vi "Process.vi"(8 "error in":errorcluster, 11 "Control Experiment":refnum<class "SMO.Control Experiment.lvclass">) -> (0 "error out":errorcluster, 3 "Control Experiment out":refnum<class "SMO.Control Experiment.lvclass">)   [LabVIEW 2019, in "SMO.Control Experiment.lvclass"]
doc: "---------------------------------------------------------------\nJKI State Machine Objects™\nhttp://jki.net/state-machine-objects/\nCopyright (C) 2005-2015, JKI <info@jki.net>\nALL RIGHTS RESERVED"
uses:
  SMO.Control Experiment.lvclass
  C:/Program Files (x86)/National Instruments/LabVIEW 2019/vi.lib/JKI/JKI SMO/SMO/SMO.lvclass
  C:/Program Files (x86)/National Instruments/LabVIEW 2019/user.lib/LevyLab/Instrument Framework/SMOs/Instrument/Instrument.lvclass
  <userlib>/LevyLab/Instrument Framework/SMOs/Configuration/Configuration.lvclass
  SMO.Control Experiment UI/Typedefs/UI Config--Cluster.ctl
  SMO.Control Experiment UI/Typedefs/UI Channels--Cluster.ctl
  SMO.Control Experiment UI/Typedefs/UI Channels.AI--Cluster.ctl
  SMO.Control Experiment UI/Typedefs/UI Channels.Device--Cluster.ctl
  Control Experiment/Typedefs/KH Mode-enum.ctl
  SMO.Control Experiment UI/Typedefs/UI Channels.KH--Cluster.ctl
  <userlib>/LevyLab/Krohn Hite 7008/typedefs/Input Configuration-Enum.ctl
  <userlib>/LevyLab/Krohn Hite 7008/typedefs/Gain-Enum.ctl
  <userlib>/LevyLab/Krohn Hite 7008/typedefs/Shunt-Enum.ctl
  SMO.Control Experiment UI/Typedefs/UI Channels.AO--Cluster.ctl
  Control Experiment/Typedefs/Instrument--enum.ctl
  <userlib>/LevyLab/Krohn Hite 7008/typedefs/Coupling-Enum.ctl
  <userlib>/LevyLab/Krohn Hite 7008/typedefs/Filter-Enum.ctl
  SMO.Control Experiment UI/Typedefs/KH Cluster--Cluster.ctl
  <userlib>/LevyLab/Krohn Hite 7008/typedefs/SetAll-Cluster.ctl
  <userlib>/LevyLab/Krohn Hite 7008/typedefs/Channel-Enum.ctl
  SMO.Control Experiment.lvclass/SMO.Control Experiment.ctl
  <vilib>/JKI/JKI SMO/SMO/SMO.lvclass/SMO.ctl
  <vilib>/Utility/sysdir.llb/System Directory Type.ctl
  Control Experiment/Typedefs/Experiment Description--cluster.ctl
  Control Experiment/Typedefs/Instrument Types--combo.ctl
  Control Experiment/Control Experiment.lvclass/Control Experiment.ctl
  Control Experiment/Typedefs/Wiring Description--v2--cluster.ctl
  Control Experiment/Typedefs/Control Experiment JSON--cluster.ctl
  <userlib>/LevyLab/Krohn Hite 7008/Instrument.KH7008.lvclass/Instrument.KH7008.ctl
  c232f248-acab-4811-9a90-d7a35ba50f8f.vi
  <vilib>/JKI/JKI SMO/SMO/Private/ReftoDVR--SMO.vi
  <vilib>/JDP Science/JSONtext/Variant to JSON Text.vi
  <vilib>/JDP Science/JSONtext/LVClass Serializer/JSONtext LVClass Serializer.lvclass
  <userlib>/LevyLab/Instrument Framework/SMOs/Instrument/Instrument.lvclass
  <userlib>/LevyLab/Krohn Hite 7008/Instrument.KH7008.lvclass
  <userlib>/LevyLab/Lockin-Multichannel/Instrument.Lockin/Instrument.Lockin.lvclass
  <userlib>/LevyLab/Instrument Framework/Instrument Types/Strain/Instrument.Strain.lvclass
  <userlib>/LevyLab/Instrument Framework/Instrument Types/CBridge/Instrument.CBridge.lvclass
  <vilib>/JKI/JKI SMO/SMO/SMO.lvclass
  Control Experiment/Control Experiment.lvclass
  SMO.Control Experiment UI/SMO.Control Experiment UI.lvclass
panel:
  # "Instrument.\nControl Experiment\nBackend"
  # "For instructions on how to use the JKI State Machine Objects, examples and video tutorials, visit:\nhttp://jki.net/state-machine-objects/\n\nJKI State Machine Objects™\nhttp://jki.net/state-machine-objects/\nCopyright (C) 2005-2015, JKI <info@jki.net>\nALL RIGHTS RESERVED"
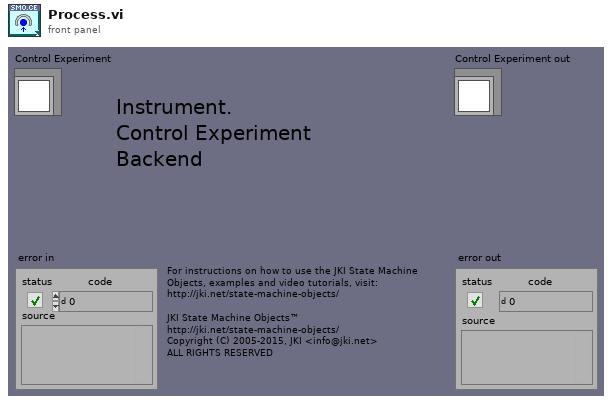
[diagram p1: front panel]
types:
  T1 = enum32{"invalid app kind", "Development System", "Run Time System", "Student Edition", "Embedded LabVIEW", "Evaluation", "Custom"}
  T2 = enum32{"Invalid", "Standard", "Closed", "Hidden", "Minimized", "Maximized"}
  T3 = enum32{"Bad", "Idle", "Run top level", "Running"}
  T4 = typedef "Control Experiment.lvclass/Experiment Description--cluster.ctl" = cluster{"User":string, "Device":string, "Device Path":path, "Device Description":string, "Experiment Path":path, "Experiment Description":string, "Instrument":T5, "Instruments":cluster{"class path":path, "Address":string, "Type":T6}[], "Sweep":cluster{"key":string, "value":variant}[]}
  T5 = typedef "Control Experiment.lvclass/Instrument--enum.ctl" = enum16{"----- AFM/EBL -----", "AGILENT", "CYPHER", "Gemini2", "JEOL", "MFP3D", "----- Cryostat -----", "CF900", "DR200", "MNK", "PPMS (simulated)", "PPMS 1", "PPMS 2", "PPMS 3", "----- Optics -----", "THz 1 (Element 2/Montana)", "THz 2 (Tsunami/Janis)"}
  T6 = typedef "Control Experiment.lvclass/Instrument Types--combo.ctl" = string
  T7 = typedef "Control Experiment.lvclass/Wiring Description--v2--cluster.ctl" = cluster{"AI":cluster{"Channel":u32, "Gain":dbl}, "Device":cluster{"Electrode":string, "Label":string, "Type":string}, "KH":cluster{"Channel":string, "Configuration":string, "Gain":u32, "Shunt Resistor":u32}, "AO":cluster{"Channel":u32, "Gain":dbl}}
  T8 = typedef "SMO.Control Experiment.lvclass/PrivateEvents--Control Experiment.saveKHpreset.ctl" = string
  T9 = typedef "SMO.Control Experiment.lvclass/PrivateEvents--Control Experiment.loadKHpreset.ctl" = string
  T10 = typedef "SMO.Control Experiment.lvclass/UI Config--Cluster.ctl" = cluster{"Metadata":cluster{"Sample (SAXXXX)":string, "Device (YYYYMMDD)":string, "Description":string, "Username":string, "Default Path":path}, "Number of AI":i32, "UI Channels []":T11[], "Instruments":cluster{"Lockin Address":string, "Krohn Hite?":bool, "KH Addresses":refnum<visa-resource-name>[], "Strain Cell?":bool, "Strain Cell Address":refnum<visa-resource-name>, "C Bridge?":bool, "Capacitance Bridge Address":refnum<visa-resource-name>, "Instrument":T5}, "Krohn Hite":cluster{"Defualt Shunt Resistor":T18, "Default Gain":T17, "Coupling":T20, "Bandwidth Filter":T21}}
  T11 = typedef "SMO.Control Experiment UI.lvclass/UI Channels--Cluster.ctl" = cluster{"AI":T12, "Device":T13, "KH":T15, "AO":T19}
  T12 = typedef "SMO.Control Experiment UI.lvclass/UI Channels.AI--Cluster.ctl" = cluster{"Channel":u32, "Gain":dbl}
  T13 = typedef "SMO.Control Experiment UI.lvclass/UI Channels.Device--Cluster.ctl" = cluster{"Electrode":string, "Configuration":T14, "Label":u16}
  T14 = typedef "Control Experiment.lvclass/KH Mode-enum.ctl" = enum16{"Ground", "Current", "Voltage (SE)", "Voltage (Diff)", "Gate"}
  T15 = typedef "SMO.Control Experiment UI.lvclass/UI Channels.KH--Cluster.ctl" = cluster{"Channel":u16, "Configuration":T16, "Gain":T17, "Shunt Resistor":T18}
  T16 = typedef "Instrument.KH7008.lvclass/Input Configuration-Enum.ctl" = enum16{"Ground", "SE+ (-gnd)", "SE- (+gnd)", "Differential"}
  T17 = typedef "Instrument.KH7008.lvclass/Gain-Enum.ctl" = enum16{"1x", "10x", "100x", "1000x"}
  T18 = typedef "Instrument.KH7008.lvclass/Shunt-Enum.ctl" = enum16{"Open", "50 Ohms", "500 Ohms", "5k Ohms", "50k Ohms", "10M Ohm"}
  T19 = typedef "SMO.Control Experiment UI.lvclass/UI Channels.AO--Cluster.ctl" = cluster{"Channel":u32, "Gain":dbl}
  T20 = typedef "Instrument.KH7008.lvclass/Coupling-Enum.ctl" = enum16{"AC", "DC"}
  T21 = typedef "Instrument.KH7008.lvclass/Filter-Enum.ctl" = enum16{"OFF", "ON"}
  T22 = typedef "SMO.Control Experiment UI.lvclass/KH Cluster--Cluster.ctl" = cluster{"VISA Resource Name":refnum<visa-resource-name>, "KH Ch Array":T23[]}[]
  T23 = typedef "Instrument.KH7008.lvclass/SetAll-Cluster.ctl" = cluster{"Channel":T24, "Gain":T17, "Bandwidth Filter":T21, "Shunt Resistor":T18, "Coupling":T20, "Input Config":T16}
  T24 = typedef "Instrument.KH7008.lvclass/Channel-Enum.ctl" = enum16{"Channel 1", "Channel 2", "Channel 3", "Channel 4", "Channel 5", "Channel 6", "Channel 7", "Channel 8"}
  T25 = cluster{"Core":cluster{"Current VI Reference":refnum<vi>, "Close Panel on Exit?":bool, "error":errorcluster}, "Self Reference":refnum<class "SMO.Control Experiment.lvclass">, "C.E.":refnum<class "Control Experiment.lvclass">, "Config":refnum<class "Configuration.lvclass">, "UI Config":T10, "KH Cluster":T22}
  T26 = cluster{"Current VI Reference":refnum<vi>, "Close Panel on Exit?":bool, "error":errorcluster}
  T27 = typedef "SMO.lvclass/Protected Events.ctl" = cluster{"StopProcesses":refnum<user-event>, "AbortProcesses":refnum<user-event>, "Config Changed":refnum<user-event>, "Dependency":refnum<user-event>}
  T28 = typedef "SMO.Control Experiment.lvclass/PrivateEvents--Cluster.ctl" = cluster{"saveKHpreset":refnum<user-event>, "setUIconfig":refnum<user-event>, "loadKHpreset":refnum<user-event>}
  T29 = typedef "System Directory Type.ctl" = i32
  T30 = typedef "Control Experiment.lvclass/Control Experiment JSON--cluster.ctl" = cluster{"Device":cluster{"Device":string, "User":string, "Time":string, "Computer Name":string}, "Wiring":cluster{"Lockin Ch":u32[], "KH Electrodes":string[], "KH Labels":string[], "Other Electrodes":string[], "Other Labels":string[]}}
  T31 = typedef "Control Experiment.lvclass/Instruments--cluster.ctl" = cluster{"KH7008":refnum<class "Instrument.KH7008.lvclass">[], "Lockin":refnum<class "Instrument.Lockin.lvclass">, "Temperature":refnum<class "Instrument.Cryostat.lvclass">, "Magnet":refnum<class "Instrument.Cryostat.lvclass">, "Rotator":refnum<class "Instrument.Cryostat.lvclass">, "Level":refnum<class "Instrument.Cryostat.lvclass">, "Capacitance Bridge":refnum<class "Instrument.CBridge.lvclass">, "Delay Line":refnum<class "Instrument.DelayLine.lvclass">, "Strain Cell":refnum<class "Instrument.Strain.lvclass">, "VNA":refnum<class "Instrument.VNA.lvclass">, "Voltage Source":refnum<class "Instrument.VSource.lvclass">}
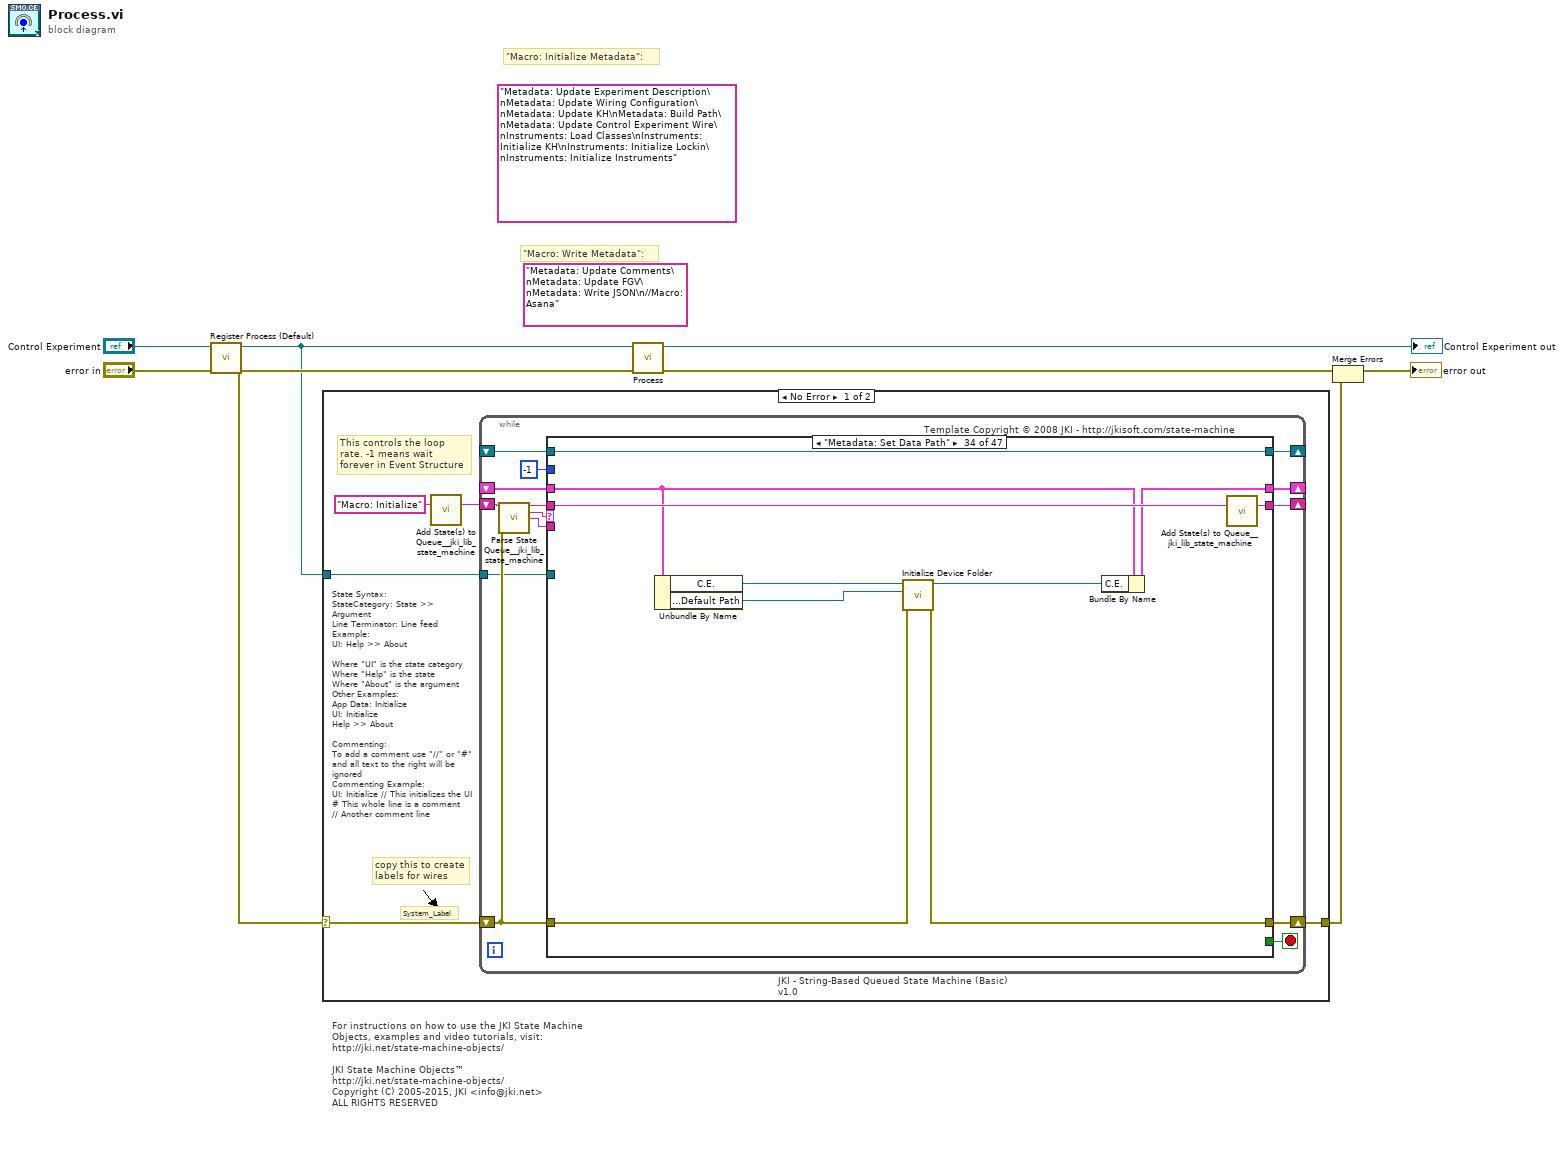
[diagram p0: block diagram]
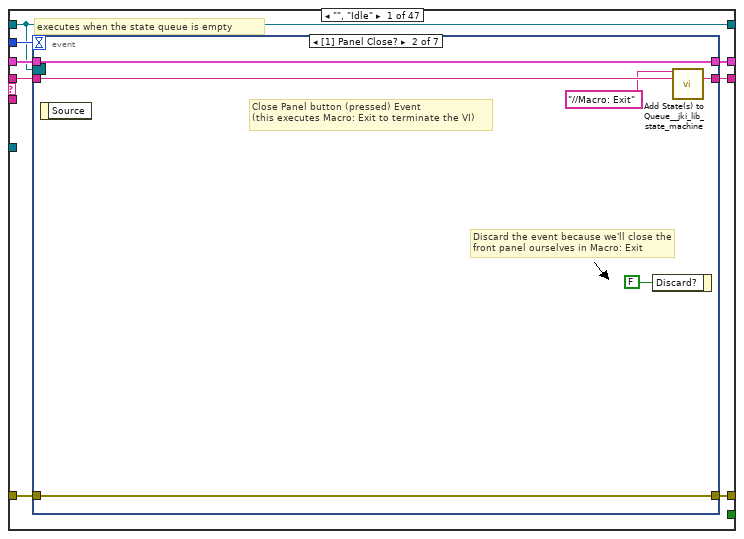
[diagram p2: hidden frame]
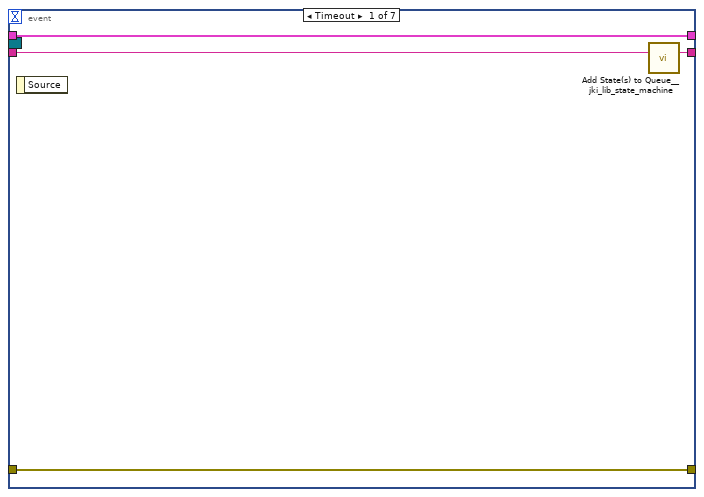
[diagram p3: hidden frame]
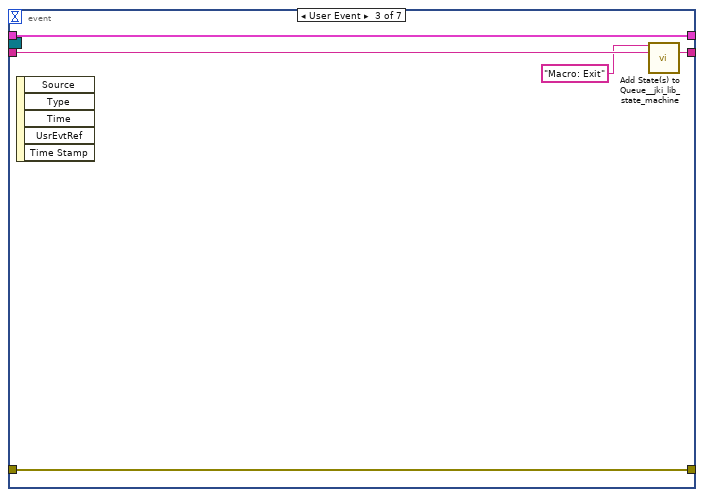
[diagram p4: hidden frame]
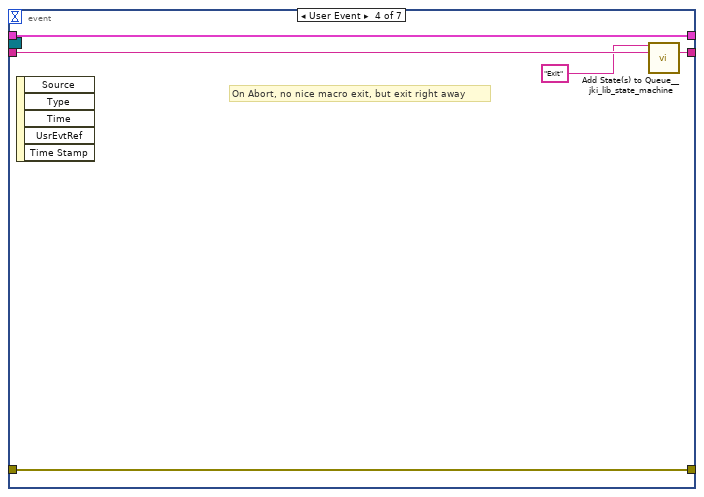
[diagram p5: hidden frame]
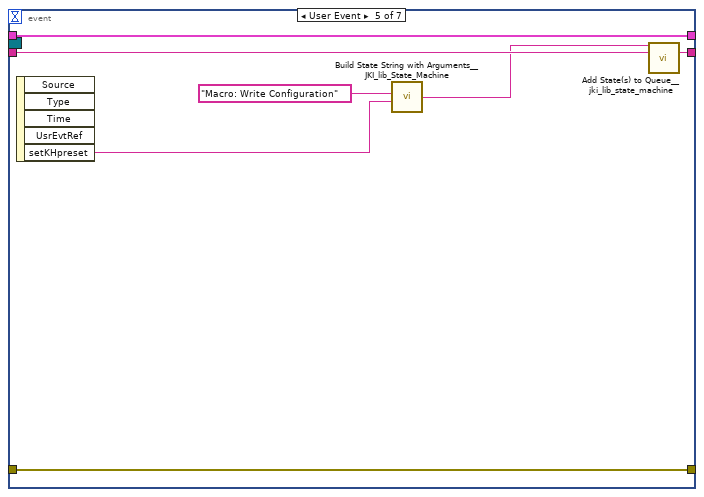
[diagram p6: hidden frame]
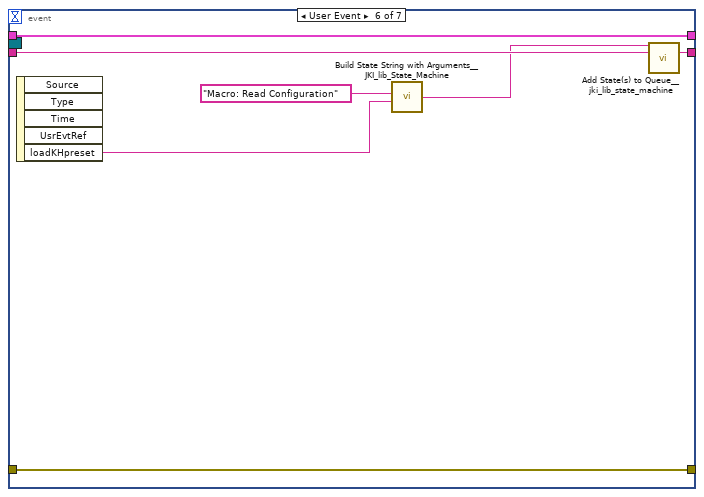
[diagram p7: hidden frame]
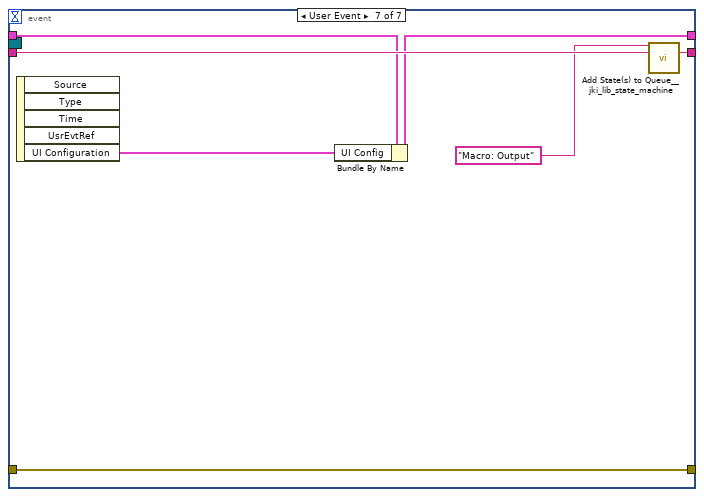
[diagram p8: hidden frame]
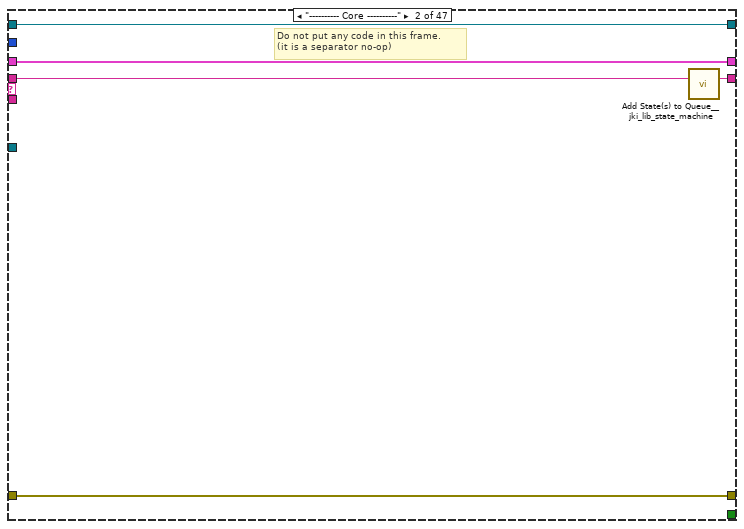
[diagram p9: hidden frame]
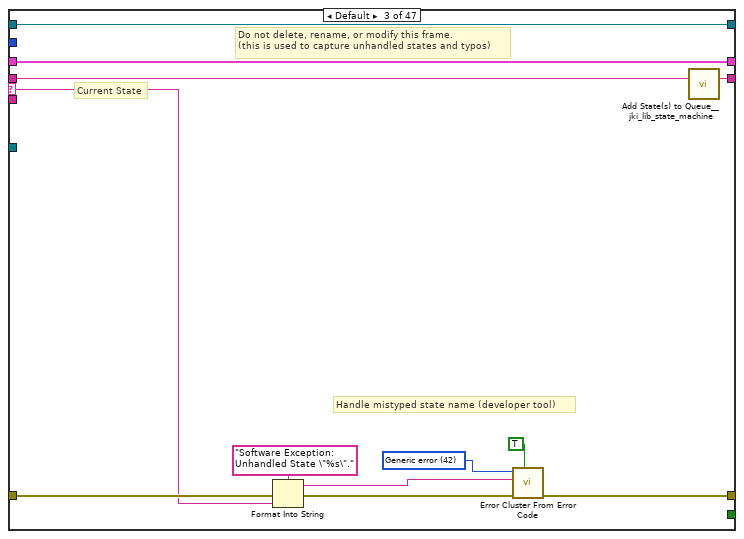
[diagram p10: hidden frame]
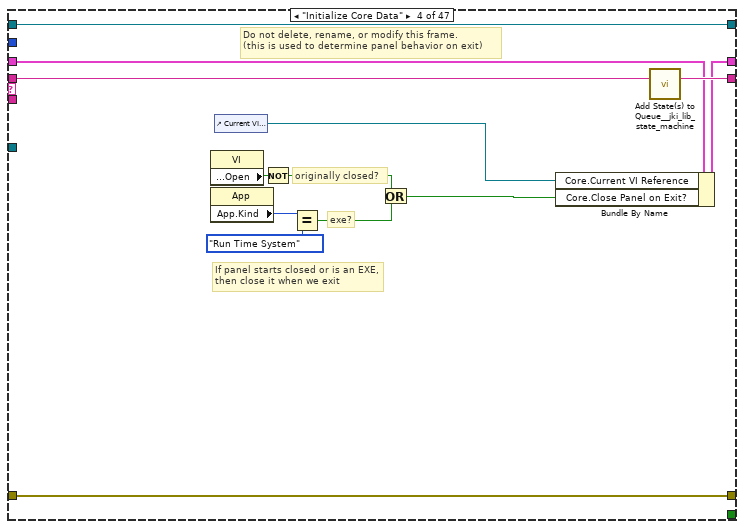
[diagram p11: hidden frame]
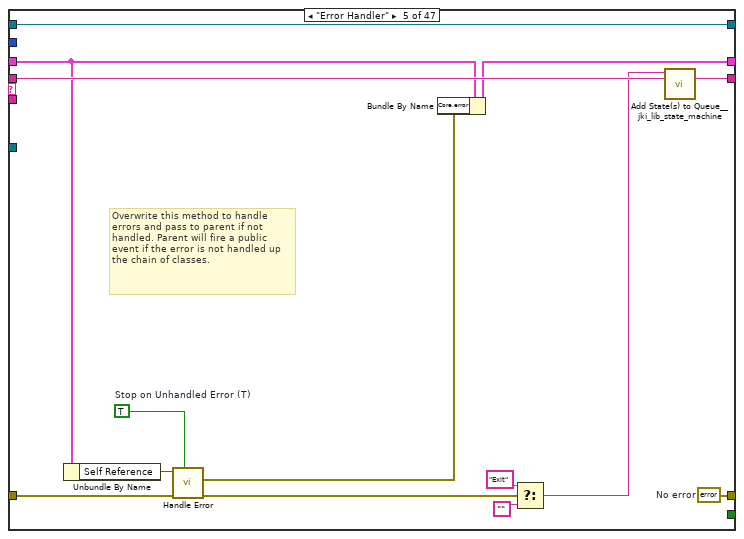
[diagram p12: hidden frame]
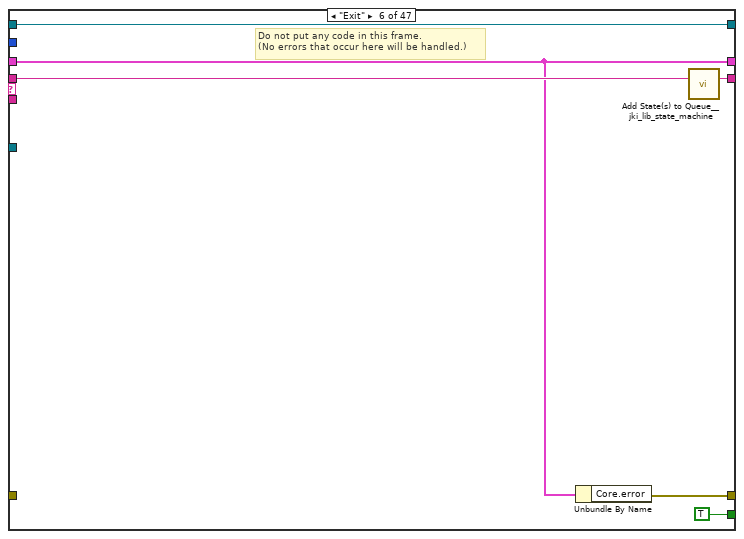
[diagram p13: hidden frame]
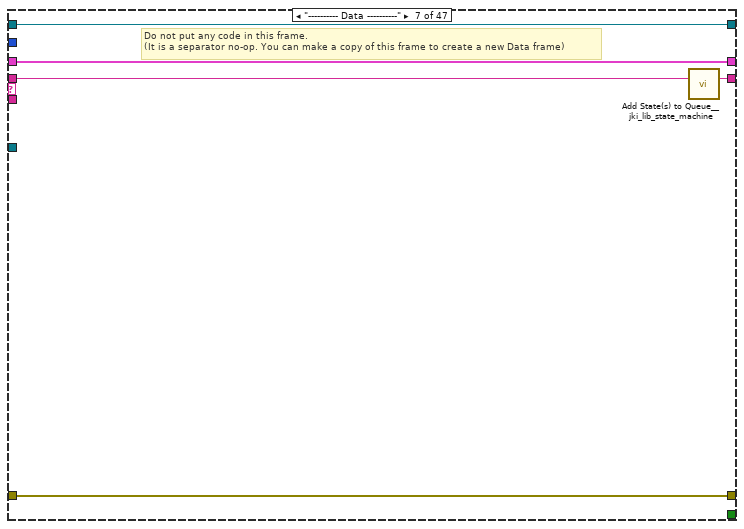
[diagram p14: hidden frame]
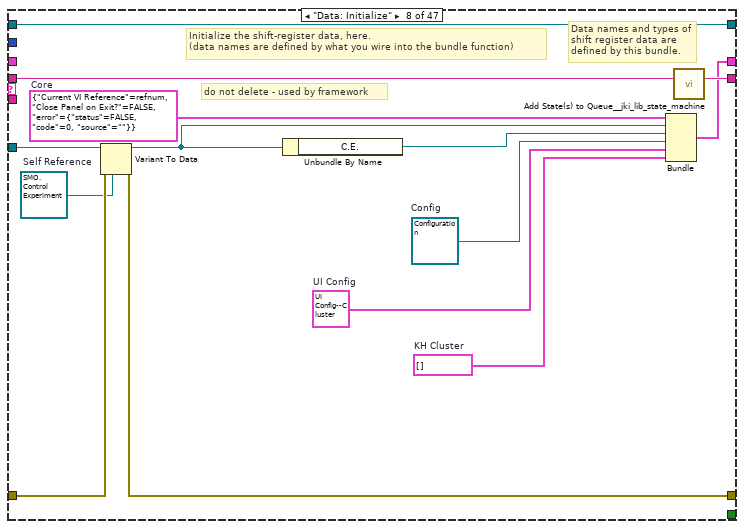
[diagram p15: hidden frame]
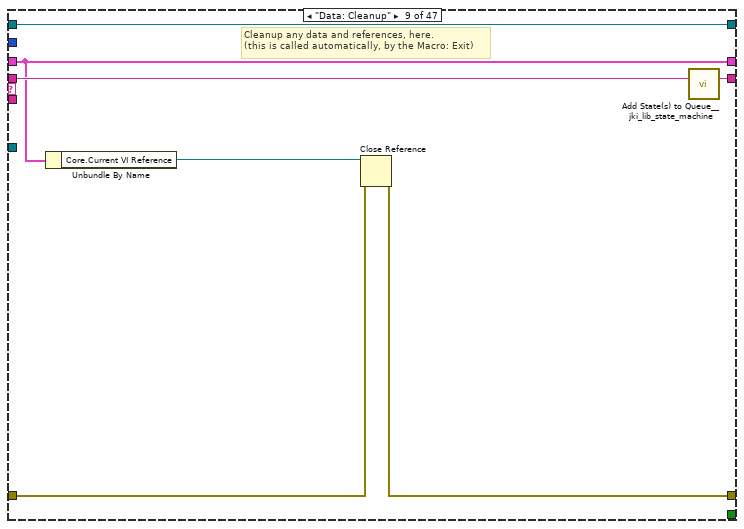
[diagram p16: hidden frame]
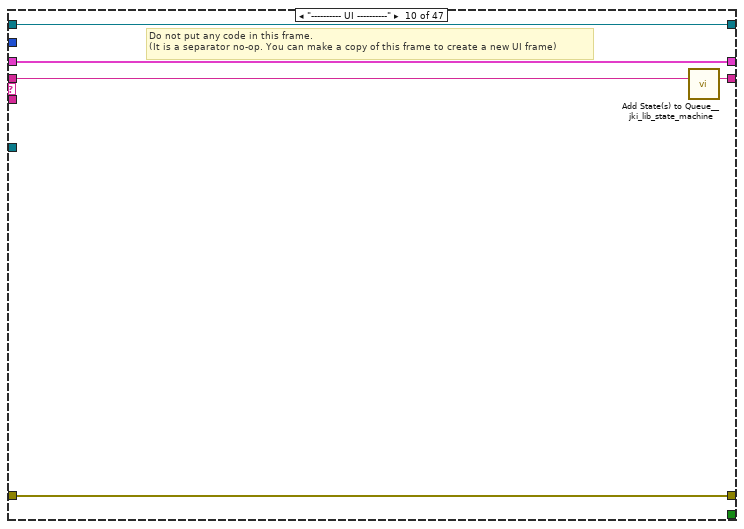
[diagram p17: hidden frame]
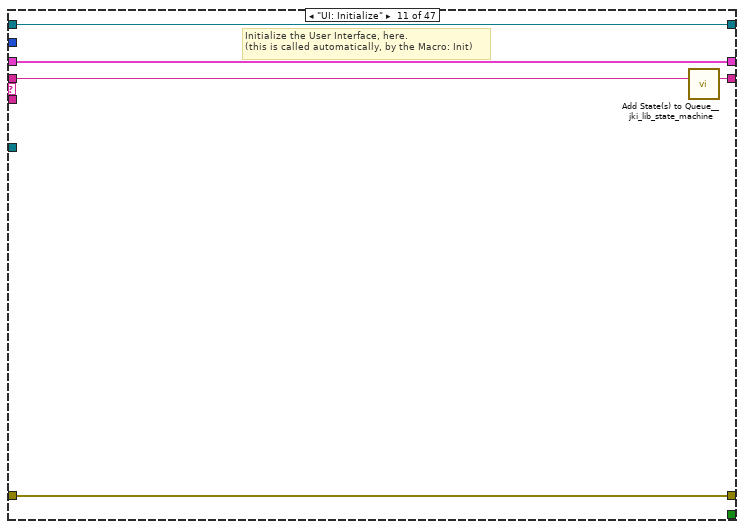
[diagram p18: hidden frame]
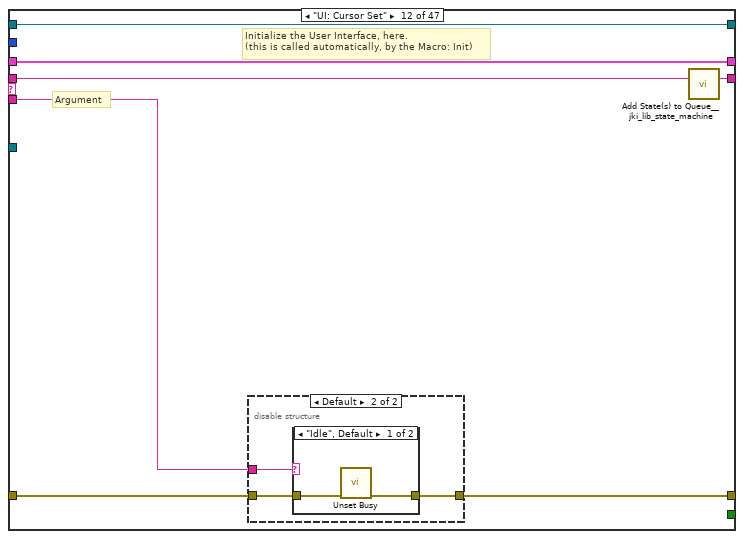
[diagram p19: hidden frame]
diagram:
  (unwired) "Metadata: Update Comments\nMetadata: Update FGV\nMetadata: Write JSON\n//Macro: Asana" ("State(s) in Front (\"\")")
  (unwired) "Metadata: Update Experiment Description\nMetadata: Update Wiring Configuration\nMetadata: Update KH\nMetadata: Build Path\nMetadata: Update Control Experiment Wire\nInstruments: Load Classes\nInstruments: Initialize KH\nInstruments: Initialize Lockin\nInstruments: Initialize Instruments" ("State(s) in Front (\"\")")
  # "\"Macro: Write Metadata\":"
  # "\"Macro: Initialize Metadata\":"
  # "For instructions on how to use the JKI State Machine Objects, examples and video tutorials, visit:\nhttp://jki.net/state-machine-objects/\n\nJKI State Machine Objects™\nhttp://jki.net/state-machine-objects/\nCopyright (C) 2005-2015, JKI <info@jki.net>\nALL RIGHTS RESERVED"
  n1 = call <vilib>:"Register Process (Default).vi"("error in (no error)"="error in", "SMO"="Control Experiment") -> ("error out"=w5:errorcluster, "SelfRef"=w4:refnum<class "SMO.Control Experiment.lvclass">)  [unwired: 8 in]
  n2 = case shown="No Error" w5 {
    selector: w5 -> [w10 w693]
    tunnel: w4 -> [w11 _]
    tunnel: [w9 w693] -> w1
    frame No Error {
      # "State Syntax:\nStateCategory: State >> Argument\nLine Terminator: Line feed\nExample:\nUI: Help >> About\n\nWhere \"UI\" is the state category\nWhere \"Help\" is the state\nWhere \"About\" is the argument\nOther Examples:\nApp Data: Initialize\nUI: Initialize\nHelp >> About\n\nCommenting:\nTo add a comment use \"//\" or \"#\" and all text to the right will be ignored\nCommenting Example:\nUI: Initialize // This initializes the UI\n# This whole line is a comment\n// Another comment line"
      # "copy this to create labels for wires"
      # "This controls the loop rate. -1 means wait forever in Event Structure"
      # "System_Label"
      n3 = call <vilib>:"Add State(s) to Queue__jki_lib_state_machine.vi"("State(s) in (\"\")"="Macro: Initialize") -> ("States Out"=w13:string)  [unwired: 14 in]
      n4 = while "JKI - String-Based Queued State Machine (Basic) v1.0" {
        shift-right: [w20] -> _
        shift-left: _ -> [w19]
        shift-right: [w23] -> w9
        shift-left: w10 -> [w17]
        shift-right: [w22] -> _
        shift-left: w13 -> [w24]
        tunnel: w11 -> [w16]
        shift-right: [w15] -> _
        shift-left: _ -> [w14]
        stop <- w21 stop-if-true
        # "Template Copyright © 2008 JKI - http://jkisoft.com/state-machine"
        n5 = call <vilib>:"Parse State Queue__jki_lib_state_machine.vi"("State Queue"=w24, "Error In (no error)"=w17) -> ("Remaining States"=w26:string, "Current State"=w27:string, "Arguments"=w25:string)  [unwired: 11 in]
        n6 = case shown="\"Metadata: Set Data Path\"" w27 {
          selector: w27 -> [_ _ w83 _ _ _ _ _ _ _ _ _ _ _ _ _ _ _ _ _ _ _ _ _ _ _ _ _ _ _ _ _ _ _ _ _ _ _ _ _ _ _ _ _ _ _ _]
          tunnel: w26 -> [w35 w81 w87 w106 w120 w126 w131 w145 w152 w157 w162 w169 w185 w217 w240 w250 w260 w269 w290 w295 w306 w311 w324 w330 w335 w353 w367 w375 w380 w385 w392 w410 w421 w461 w472 w497 w506 w515 w533 w555 w567 w592 w623 w641 w659 w669 w692]
          tunnel: w25 -> [_ _ _ _ _ _ _ _ _ _ _ w163 w179 _ _ w242 w252 _ _ _ _ _ _ _ _ w339 _ _ _ _ _ _ _ _ _ _ _ _ _ _ _ _ _ _ _ _ _]
          tunnel: w19 -> [w33 w78 w85 w97 w114 w122 w128 _ w147 w154 w160 w167 w181 w214 w237 w247 w257 w266 w271 w292 w303 w308 w316 w328 w333 w338 w359 w370 w378 w383 w387 w407 w417 w457 w468 w493 w501 w511 w529 w551 w562 w589 w619 w637 w655 w665 w688]
          tunnel: [w32 w79 w89 w103 w115 w121 w129 w137 w148 w155 w159 w164 w182 w215 w219 w248 w258 w267 w273 w293 w297 w309 w319 w326 w331 w340 w355 w368 w376 w381 w389 w400 w413 w454 w462 w475 w503 w507 w524 w542 w556 w578 w614 w632 w650 w660 w680] -> w23
          tunnel: w17 -> [w31 w79 w88 w103 w116 _ w129 w142 w149 w155 w159 w165 w183 w215 w220 w248 w258 w267 w274 w293 w298 w309 w320 w326 w331 w341 w360 w369 w376 w381 w389 w401 w414 w455 w463 w483 w503 w508 w522 w543 w563 w571 w611 w629 w647 w661 w681]
          tunnel: [w34 w80 w86 w105 w119 w125 w130 w144 w151 w156 w161 w168 w184 w216 w239 w249 w259 w268 w289 w294 w305 w310 w323 w329 w334 w352 w366 w374 w379 w384 w391 w409 w420 w460 w471 w496 w505 w514 w532 w554 w566 w591 w622 w640 w658 w668 w691] -> w22
          tunnel: [_ _ _ _ _ TRUE _ _ _ _ _ _ _ _ _ _ _ _ _ _ _ _ _ _ _ _ _ _ _ _ _ _ _ _ _ _ _ _ _ _ _ _ _ _ _ _ _] -> w21
          tunnel: [w30 w78 w85 w104 w113 w122 w128 w143 w147 w154 w160 w167 w181 w214 w237 w247 w257 w266 w271 w292 w303 w308 w316 w328 w333 w337 w358 w370 w378 w383 w388 w406 w418 w458 w469 w494 w502 w512 w530 w552 w562 w589 w620 w638 w656 w666 w689] -> w20
          tunnel: -1 ("Timeout") -> [w29 _ _ _ _ _ _ _ _ _ _ _ _ _ _ _ _ _ _ _ _ _ _ _ _ _ _ _ _ _ _ _ _ _ _ _ _ _ _ _ _ _ _ _ _ _ _]
          tunnel: w16 -> [_ _ _ _ _ _ _ w140 _ _ _ _ _ _ w228 _ _ _ w270 _ _ _ _ _ _ _ _ _ _ _ _ _ _ _ _ _ _ _ _ _ _ _ _ _ _ _ _]
          tunnel: [w28 w77 w82 w94 w118 w123 w127 w139 w146 w153 w158 w166 w178 w213 w238 w246 w256 w265 w284 w291 w304 w307 w322 w327 w332 w351 w365 w373 w377 w382 w390 w408 w419 w459 w470 w495 w504 w513 w531 w553 w565 w590 w621 w639 w657 w667 w690] -> w15
          tunnel: w14 -> [w28 w77 w82 w94 w118 w123 w127 w139 w146 w153 w158 w166 w178 w213 w238 w246 w256 w265 w284 w291 w304 w307 _ w327 w332 w351 w365 w373 w377 w382 w390 w408 w419 w459 w470 w495 w504 w513 w531 w553 w565 w590 w621 w639 w657 w667 w690]
          frame "", "Idle" {
            # "executes when the state queue is empty"
            n7 = event shown="[1] Panel Close?" {
              selector: w28 -> [_ _ _ _ _ _ _]
              dyn-events: _ -> [_ _ _ _ _ _ _]
              timeout: w29 -> [_ _ _ _ _ _ _]
              tunnel: w35 -> [w39 w45 w50 w55 w62 w69 w76]
              tunnel: [w38 w44 w49 w54 w61 w68 w75] -> w34
              tunnel: w33 -> [w36 w42 w47 w52 w59 w66 w73]
              tunnel: [w37 w43 w48 w53 w60 w67 w74] -> w32
              tunnel: w31 -> [w37 w43 w48 w53 w60 w67 w74]
              tunnel: [w36 w42 w47 w52 w59 w66 w72] -> w30
              event Timeout {
                n8 = event-data() -> ()  [unwired: 1 in, 1 out]
                n9 = call <vilib>:"Add State(s) to Queue__jki_lib_state_machine.vi"("State(s) in (\"\")"=w39) -> ("States Out"=w38:string)  [unwired: 14 in]
              }
              event Panel Close? {
                # "Discard the event because we'll close the front panel ourselves in Macro: Exit"
                # "Close Panel button (pressed) Event\n(this executes Macro: Exit to terminate the VI)"
                n10 = event-data() -> ()  [unwired: 1 in, 1 out]
                n11 = event-data("Discard?"=FALSE) -> ()  [unwired: 1 in, 1 out]
                n12 = call <vilib>:"Add State(s) to Queue__jki_lib_state_machine.vi"("State(s) in Front (\"\")"="//Macro: Exit", "State(s) in (\"\")"=w45) -> ("States Out"=w44:string)  [unwired: 13 in]
              }
              event User Event {
                n13 = event-data() -> ()  [unwired: 1 in, 5 out]
                n14 = call <vilib>:"Add State(s) to Queue__jki_lib_state_machine.vi"("State(s) in Front (\"\")"="Macro: Exit", "State(s) in (\"\")"=w50) -> ("States Out"=w49:string)  [unwired: 13 in]
              }
              event User Event {
                # "On Abort, no nice macro exit, but exit right away"
                n15 = event-data() -> ()  [unwired: 1 in, 5 out]
                n16 = call <vilib>:"Add State(s) to Queue__jki_lib_state_machine.vi"("State(s) in Front (\"\")"="Exit", "State(s) in (\"\")"=w55) -> ("States Out"=w54:string)  [unwired: 13 in]
              }
              event User Event {
                n17 = event-data() -> ("setKHpreset"=w56:T8)  [unwired: 1 in, 4 out]
                n18 = call <vilib>:"Build State String with Arguments__JKI_lib_State_Machine.vi"("Arguments (\"\")"=w56, "State"="Macro: Write Configuration" ("State(s) in Front (\"\")")) -> ("State with Arguments"=w57:string)  [unwired: 4 in]
                n19 = call <vilib>:"Add State(s) to Queue__jki_lib_state_machine.vi"("State(s) in Front (\"\")"=w57, "State(s) in (\"\")"=w62) -> ("States Out"=w61:string)  [unwired: 13 in]
              }
              event User Event {
                n20 = event-data() -> ("loadKHpreset"=w63:T9)  [unwired: 1 in, 4 out]
                n21 = call <vilib>:"Build State String with Arguments__JKI_lib_State_Machine.vi"("Arguments (\"\")"=w63, "State"="Macro: Read Configuration" ("State(s) in Front (\"\")")) -> ("State with Arguments"=w64:string)  [unwired: 4 in]
                n22 = call <vilib>:"Add State(s) to Queue__jki_lib_state_machine.vi"("State(s) in Front (\"\")"=w64, "State(s) in (\"\")"=w69) -> ("States Out"=w68:string)  [unwired: 13 in]
              }
              event User Event {
                n23 = event-data() -> ("UI Configuration"=w71:T10)  [unwired: 1 in, 4 out]
                n24 = Bundle By Name(cluster=w73, "UI Config"=w71) -> (w72:T25)
                n25 = call <vilib>:"Add State(s) to Queue__jki_lib_state_machine.vi"("State(s) in Front (\"\")"="Macro: Output" ("State(s) in Front (\"\")"), "State(s) in (\"\")"=w76) -> ("States Out"=w75:string)  [unwired: 13 in]
              }
            }
          }
          frame "---------- Core ----------" {
            # "Do not put any code in this frame.\n(it is a separator no-op)"
            n26 = call <vilib>:"Add State(s) to Queue__jki_lib_state_machine.vi"("State(s) in (\"\")"=w81) -> ("States Out"=w80:string)  [unwired: 14 in]
          }
          frame Default {
            w92 = 42 items=["No error", "Argument error", "Memory is full", "Out of zone", "End of file", "File already open", "Generic file I/O error", "File not found", "File permission error", "Disk is full", "Duplicate path", "Too many files open", "System feature not enabled", "Resource file not found", "Cannot add resource", "Resource not found", "Image not found", "Image memory error", "Pen does not exist", "Config type invalid", "Config token not found", "Config parse error", "Config memory error", "Bad external code format", "Bad external code offset", "External code not present", "Null window", "Destroy window error", "Null menu", "Print aborted", "Bad print record", "Print driver error", "Windows error during printing", "Memory error during printing", "Print dialog error", "Generic print error", "Invalid device refnum", "Device not found", "Device parameter error", "Device unit error", "Cannot open device", "Device call aborted", "Generic error", "Cancelled by user", "Object ID too low", "Object ID too high", "Object not in heap", "Unknown heap", "Unknown object (invalid DefProc)", "Unknown object (DefProc not in table)", "Message out of range", "Invalid (null) method", "Unknown message", "Manager call not supported", "Bad address", "Network operation in progress", "Network operation timed out", "Connection is busy", "Network attribute not supported", "Network error", "Address in use", "System out of memory", "Connection aborted", "Connection refused", "Not connected", "Already connected", "Connection closed", "Initialization error (interapplication manager)", "Bad occurrence", "Wait on unbound occurrence handler", "Occurrence queue overflow", "Datalog type conflict", "Unused", "Unrecognized type (interapplication manager)", "Memory corrupt", "Failed to make temporary DLL", "Old CIN version", "Drag socket not found", "Failed to load drop-object", "Failed to register OLE object", "Failed to release OLE object", "Format specifier type mismatch", "Unknown format specifier", "Too few format specifiers", "Too many format specifiers", "Scan failed", "Newer CIN version", "Error converting to variant", "Runtime menu error", "Password tampered", "Variant attribute not found", "Incompatible variant data type", "Event data is not available", "Event Store is not present", "Occurrence is not found", "Event Queue is not created", "Event info is not available", "Refnum passed is NULL", "Error retrieving Class GUID", "Error retrieving CoClass GUID", "Error retrieving TypeLib GUID.", "Bad built application magic bytes.", "Specific driver is different from the specific driver associated with the Logical Name.", "There is no session opened to the class driver.", "Max Error", "MAX - Error with config objects", "MAX - Error loading configuration", "MAX - Group not supported"]
            # "Current State"
            # "Do not delete, rename, or modify this frame.\n(this is used to capture unhandled states and typos)"
            # "Handle mistyped state name (developer tool)"
            n27 = Format Into String(format string="Software Exception: Unhandled State \"%s\"." ("message"), error in=w88, w83) -> (resulting string=w91:string, error out=w90:errorcluster)  [unwired: 1 in]
            n28 = call <vilib>:"Error Cluster From Error Code.vi"("show call chain? (False)"=TRUE, "error in (no error)"=w90, "error message (\"\")"=w91, "error code (0)"=w92) -> ("error out"=w89:errorcluster)  [unwired: 5 in]
            n29 = call <vilib>:"Add State(s) to Queue__jki_lib_state_machine.vi"("State(s) in (\"\")"=w87) -> ("States Out"=w86:string)  [unwired: 14 in]
          }
          frame "Initialize Core Data" {
            # "Do not delete, rename, or modify this frame.\n(this is used to determine panel behavior on exit)"
            # "originally closed?"
            # "exe?"
            # "If panel starts closed or is an EXE, then close it when we exit"
            n30 = property class="VI"() -> ("Front Panel.Open"=w102:bool)  [unwired: 2 in, 2 out]
            n31 = property class="App"() -> ("App.Kind"=w101:T1)  [unwired: 2 in, 2 out]
            n32 = control-ref of="Current VI Reference"() -> (w95:refnum<vi>)
            n33 = Not(x=w102) -> (.not. x?=w99:bool)
            n34 = Equal?(x=w101, y=T1."Run Time System" ("Application:Kind")) -> (x = y?=w98:bool)
            n35 = Or(x=w99, y=w98) -> (x .or. y?=w96:bool)
            n36 = Bundle By Name(cluster=w97, "Core.Current VI Reference"=w95, "Core.Close Panel on Exit?"=w96) -> (w104:T25)
            n37 = call <vilib>:"Add State(s) to Queue__jki_lib_state_machine.vi"("State(s) in (\"\")"=w106) -> ("States Out"=w105:string)  [unwired: 14 in]
          }
          frame "Error Handler" {
            w107 = TRUE  # Stop on Unhandled Error (T)
            w115 = errorcluster {"status"=FALSE, "code"=0, "source"=""}  # No error
            # "Overwrite this method to handle errors and pass to parent if not handled. Parent will fire a public event if the error is not handled up the chain of classes."
            n38 = Unbundle By Name(w114) -> ("Self Reference"=w117:refnum<class "SMO.Control Experiment.lvclass">)
            n39 = call-dynamic "Handle Error.vi"("Stop on Unhandled Error (T)"=w107, "error in"=w116, "SMO"=w117) -> ("handling error"=w108:errorcluster, "Unhandled error"=w111:errorcluster)  [unwired: 6 in, 1 out]
            n40 = Bundle By Name(cluster=w114, "Core.error"=w111) -> (w113:T25)
            n41 = Select(t="Exit", s=w108, f="") -> (s? t:f=w112:string)
            n42 = call <vilib>:"Add State(s) to Queue__jki_lib_state_machine.vi"("State(s) in Front (\"\")"=w112, "State(s) in (\"\")"=w120) -> ("States Out"=w119:string)  [unwired: 13 in]
          }
          frame "Exit" {
            # "Do not put any code in this frame.\n(No errors that occur here will be handled.)"
            n43 = Unbundle By Name(w122) -> ("Core.error"=w121:errorcluster)
            n44 = call <vilib>:"Add State(s) to Queue__jki_lib_state_machine.vi"("State(s) in (\"\")"=w126) -> ("States Out"=w125:string)  [unwired: 14 in]
          }
          frame "---------- Data ----------" {
            # "Do not put any code in this frame.\n(It is a separator no-op. You can make a copy of this frame to create a new Data frame)"
            n45 = call <vilib>:"Add State(s) to Queue__jki_lib_state_machine.vi"("State(s) in (\"\")"=w131) -> ("States Out"=w130:string)  [unwired: 14 in]
          }
          frame "Data: Initialize" {
            w134 = T22 []  # KH Cluster
            w135 = T10 {"Metadata"={"Sample (SAXXXX)"="", "Device (YYYYMMDD)"="", "Description"="", "Username"="", "Default Path"=path ""}, "Number of AI"=8, "UI Channels []"=[], "Instruments"={"Lockin Address"="", "Krohn Hite?"=TRUE, "KH Addresses"=[], "Strain Cell?"=TRUE, "Strain Cell Address"="", "C Bridge?"=TRUE, "Capacitance Bridge Address"="", "Instrument"=enum."----- AFM/EBL -----"}, "Krohn Hite"={"Defualt Shunt Resistor"=enum."50k Ohms", "Default Gain"=enum."10x", "Coupling"=enum."DC", "Bandwidth Filter"=enum."ON"}}  # UI Config
            w136 = refnum<class "Configuration.lvclass"> refnum  # Config
            w138 = T26 {"Current VI Reference"=refnum, "Close Panel on Exit?"=FALSE, "error"={"status"=FALSE, "code"=0, "source"=""}}  # Core
            w141 = refnum<class "SMO.Control Experiment.lvclass"> refnum  # Self Reference
            # "do not delete - used by framework"
            # "Data names and types of shift register data are defined by this bundle."
            # "Initialize the shift-register data, here.\n(data names are defined by what you wire into the bundle function)"
            n46 = Variant To Data(error in=w142, type=w141, Variant=w140) -> (data=w133:refnum<class "SMO.Control Experiment.lvclass">, error out=w137:errorcluster)
            n47 = Unbundle By Name(w133) -> ("C.E."=w132:refnum<class "Control Experiment.lvclass">)
            n48 = Bundle("Core"=w138, "Self Reference"=w133, "C.E."=w132, "Config"=w136, "UI Config"=w135, "KH Cluster"=w134) -> (w143:T25)  [unwired: 1 in]
            n49 = call <vilib>:"Add State(s) to Queue__jki_lib_state_machine.vi"("State(s) in (\"\")"=w145) -> ("States Out"=w144:string)  [unwired: 14 in]
          }
          frame "Data: Cleanup" {
            # "Cleanup any data and references, here.\n(this is called automatically, by the Macro: Exit)"
            n50 = Unbundle By Name(w147) -> ("Core.Current VI Reference"=w150:refnum<vi>)
            n51 = Close Reference(reference=w150, error in (no error)=w149) -> (error out=w148:errorcluster)
            n52 = call <vilib>:"Add State(s) to Queue__jki_lib_state_machine.vi"("State(s) in (\"\")"=w152) -> ("States Out"=w151:string)  [unwired: 14 in]
          }
          frame "---------- UI ----------" {
            # "Do not put any code in this frame.\n(It is a separator no-op. You can make a copy of this frame to create a new UI frame)"
            n53 = call <vilib>:"Add State(s) to Queue__jki_lib_state_machine.vi"("State(s) in (\"\")"=w157) -> ("States Out"=w156:string)  [unwired: 14 in]
          }
          frame "UI: Initialize" {
            # "Initialize the User Interface, here.\n(this is called automatically, by the Macro: Init)"
            n54 = call <vilib>:"Add State(s) to Queue__jki_lib_state_machine.vi"("State(s) in (\"\")"=w162) -> ("States Out"=w161:string)  [unwired: 14 in]
          }
          frame "UI: Cursor Set" {
            # "Argument"
            # "Initialize the User Interface, here.\n(this is called automatically, by the Macro: Init)"
            n55 = disable-structure shown="Default" {
              disable-tunnel: w165 -> [w170 w173]
              disable-tunnel: [w170 w172] -> w164
              disable-tunnel: w163 -> [_ w171]
              frame condition #0 {
              }
              frame condition #1 (active) {
                n56 = case shown="\"Idle\", Default" w171 {
                  tunnel: w173 -> [w175 w177]
                  tunnel: [w174 w176] -> w172
                  frame "Idle", Default {
                    n57 = call <vilib>:"Unset Busy.vi"("error in (no error)"=w175) -> ("error out"=w174:errorcluster)  [unwired: 10 in]
                  }
                  frame "Busy" {
                    n58 = call <vilib>:"Set Busy.vi"("error in (no error)"=w177) -> ("error out"=w176:errorcluster)  [unwired: 9 in, 1 out]
                  }
                }
              }
            }
            n59 = call <vilib>:"Add State(s) to Queue__jki_lib_state_machine.vi"("State(s) in (\"\")"=w169) -> ("States Out"=w168:string)  [unwired: 14 in]
          }
          frame "UI: Front Panel State" {
            # "Argument"
            # "Set Front Panel Open or Closed\n(Usage: \"UI: Front Panel State >> Open|Close\")"
            n60 = Unbundle By Name(w181) -> ("Core.Current VI Reference"=w180:refnum<vi>)
            n61 = disable-structure shown="Default" {
              disable-tunnel: w183 -> [w189 w212]
              disable-tunnel: [w188 w212] -> w182
              disable-tunnel: w180 -> [w187 _]
              disable-tunnel: w179 -> [w186 _]
              frame condition #0 (active) {
                n62 = case shown="\"Close\"" w186 {
                  tunnel: w189 -> [w193 w206]
                  tunnel: [w195 w207] -> w188
                  tunnel: w187 -> [w194 w204]
                  frame "Open", Default {
                    n63 = property class="VI"(reference=w194, error in=w193) -> (reference out=w191:refnum<vi>, error out=w192:errorcluster, "FP.State"=w190:T2)
                    n64 = case shown="\"Closed\"" w190 {
                      tunnel: [w198 w201] -> w195
                      tunnel: w192 -> [w197 w201]
                      tunnel: w191 -> [w196 _]
                      frame "Closed" {
                        n65 = invoke class="VI" method="FP.Open"(reference=w196, error in=w197, "Activate"=TRUE, "State"=T2."Standard") -> (error out=w198:errorcluster)  [unwired: 1 in, 4 out]
                      }
                      frame Default {
                      }
                    }
                  }
                  frame "Close" {
                    n66 = property class="VI"(reference=w204, error in=w206) -> (reference out=w203:refnum<vi>, error out=w205:errorcluster, "FP.State"=w202:T2)
                    n67 = case shown="Default" w202 {
                      tunnel: [w208 w211] -> w207
                      tunnel: w205 -> [w208 w210]
                      tunnel: w203 -> [_ w209]
                      frame "Invalid", "Closed" {
                      }
                      frame Default {
                        n68 = invoke class="VI" method="FP.Close"(reference=w209, error in=w210) -> (error out=w211:errorcluster)  [unwired: 1 in, 2 out]
                      }
                    }
                  }
                }
              }
              frame condition #1 {
              }
            }
            n69 = call <vilib>:"Add State(s) to Queue__jki_lib_state_machine.vi"("State(s) in (\"\")"=w185) -> ("States Out"=w184:string)  [unwired: 14 in]
          }
          frame "---------- Macro ----------" {
            # "Do not put any code in this frame.\n(It is a separator no-op. You can make a copy of this frame to create a new Macro frame)"
            n70 = call <vilib>:"Add State(s) to Queue__jki_lib_state_machine.vi"("State(s) in (\"\")"=w217) -> ("States Out"=w216:string)  [unwired: 14 in]
          }
          frame "Macro: Initialize" {
            w229 = "Process: Sync"
            # "Initialization Macro\n(This is called once, when the VI starts)"
            n71 = control-ref of="This VI"() -> (w231:refnum<vi>)
            n72 = property class="VI"(reference=w231) -> ("Exec.State"=w230:T3)  [unwired: 1 in, 2 out]
            n73 = call-dynamic "Read Debug Mode.vi"("error in (no error)"=w220, "Instrument in"=w228) -> ("error out"=w219:errorcluster, "Debug Mode?"=w221:bool)  [unwired: 7 in, 1 out]
            n74 = Equal?(x=w230, y=T3."Run top level") -> (x = y?=w235:bool)
            n75 = Select(t="Open", s=w221, f="Close") -> (s? t:f=w226:string)
            n76 = call <vilib>:"Build State String with Arguments__JKI_lib_State_Machine.vi"("Arguments (\"\")"=w226, "State"="UI: Front Panel State") -> ("State with Arguments"=w223:string)  [unwired: 4 in]
            n77 = Select(t=w229, s=w235, f="") -> ()  [unwired: 1 out]
            n78 = call <vilib>:"Add State(s) to Queue__jki_lib_state_machine.vi"("State(s) in Front (\"\")"="UI: Initialize", "State(s) in (\"\")"=w223) -> ("States Out"=w218:string)  [unwired: 13 in]
            n79 = call <vilib>:"Add State(s) to Queue__jki_lib_state_machine.vi"("State(s) in Front (\"\")"="Data: Initialize\nInitialize Core Data\nEvents: Register", "State(s) in (\"\")"=w229, "State(s) at Back (\"\")"=w218) -> ("States Out"=w232:string)  [unwired: 12 in]
            n80 = call <vilib>:"Add State(s) to Queue__jki_lib_state_machine.vi"("State(s) in Front (\"\")"=w232, "State(s) in (\"\")"=w240) -> ("States Out"=w239:string)  [unwired: 13 in]
          }
          frame "Macro: Write Configuration" {
            # "Do not put any code in this frame.\n(It is a separator no-op. You can make a copy of this frame to create a new Macro frame)"
            n81 = call <vilib>:"Build State String with Arguments__JKI_lib_State_Machine.vi"("Arguments (\"\")"=w242, "State"="Configuration: Initialize") -> ("State with Arguments"=w243:string)  [unwired: 4 in]
            n82 = call <vilib>:"Add State(s) to Queue__jki_lib_state_machine.vi"("State(s) in Front (\"\")"=w243, "State(s) at Back (\"\")"="Configuration: Write File") -> ("States Out"=w241:string)  [unwired: 13 in]
            n83 = call <vilib>:"Add State(s) to Queue__jki_lib_state_machine.vi"("State(s) in Front (\"\")"=w241, "State(s) in (\"\")"=w250) -> ("States Out"=w249:string)  [unwired: 13 in]
          }
          frame "Macro: Read Configuration" {
            # "Do not put any code in this frame.\n(It is a separator no-op. You can make a copy of this frame to create a new Macro frame)"
            n84 = call <vilib>:"Build State String with Arguments__JKI_lib_State_Machine.vi"("Arguments (\"\")"=w252, "State"="Configuration: Initialize") -> ("State with Arguments"=w253:string)  [unwired: 4 in]
            n85 = call <vilib>:"Add State(s) to Queue__jki_lib_state_machine.vi"("State(s) in Front (\"\")"=w253, "State(s) at Back (\"\")"="Configuration: Read File") -> ("States Out"=w251:string)  [unwired: 13 in]
            n86 = call <vilib>:"Add State(s) to Queue__jki_lib_state_machine.vi"("State(s) in Front (\"\")"=w251, "State(s) in (\"\")"=w260) -> ("States Out"=w259:string)  [unwired: 13 in]
          }
          frame "Macro: Output" {
            # "Do not put any code in this frame.\n(It is a separator no-op. You can make a copy of this frame to create a new Macro frame)"
            n87 = call <vilib>:"Add State(s) to Queue__jki_lib_state_machine.vi"("State(s) in Front (\"\")"="Metadata: Set Experiment\nMetadata: Set Wiring\nMetadata: Set Data Path\n\nMetadata: Set Device JSON\n\nC.E.: Initialize Instruments\nC.E.: Open Krohn Hite\nC.E.: Open Lockin\nC.E.: Open Strain Cell\nC.E.: Open C Bridge" ("State(s) in Front (\"\")"), "State(s) in (\"\")"="C.E.: Initialize KH Cluster\nC.E.: Set Krohn Hite" ("State(s) in Front (\"\")"), "State(s) at Back (\"\")"="Metadata: Update Comments\nC.E.: Write XML\nC.E.: Write PGSQL" ("State(s) in Front (\"\")")) -> ("States Out"=w261:string)  [unwired: 12 in]
            n88 = call <vilib>:"Add State(s) to Queue__jki_lib_state_machine.vi"("State(s) in Front (\"\")"=w261, "State(s) in (\"\")"=w269) -> ("States Out"=w268:string)  [unwired: 13 in]
          }
          frame "Macro: Exit" {
            # "Exit Macro\n(This is called once, when the VI exits)"
            n89 = Unbundle By Name(w271) -> ("Core.Close Panel on Exit?"=w288:bool)
            n90 = call-dynamic "Read Debug Mode.vi"("error in (no error)"=w274, "Instrument in"=w270) -> ("error out"=w273:errorcluster, "Debug Mode?"=w272:bool)  [unwired: 7 in, 1 out]
            n91 = Select(t="Open", s=w272, f="Close") -> (s? t:f=w278:string)
            n92 = call <vilib>:"Build State String with Arguments__JKI_lib_State_Machine.vi"("Arguments (\"\")"=w278, "State"="UI: Front Panel State") -> ("State with Arguments"=w275:string)  [unwired: 4 in]
            n93 = Select(t=w275, s=w288, f="") -> (s? t:f=w286:string)
            n94 = call <vilib>:"Add State(s) to Queue__jki_lib_state_machine.vi"("State(s) in Front (\"\")"="Data: Cleanup\nEvents: Unregister", "State(s) in (\"\")"="Process: Sync", "State(s) at Back (\"\")"="Exit") -> ("States Out"=w281:string)  [unwired: 12 in]
            n95 = call <vilib>:"Add State(s) to Queue__jki_lib_state_machine.vi"("State(s) in (\"\")"=w286, "State(s) at Back (\"\")"=w281) -> ("States Out"=w285:string)  [unwired: 13 in]
            n96 = call <vilib>:"Add State(s) to Queue__jki_lib_state_machine.vi"("State(s) in Front (\"\")"=w285, "State(s) in (\"\")"=w290) -> ("States Out"=w289:string)  [unwired: 13 in]
          }
          frame "---------- Process ----------" {
            # "Template Separator\n(You can make a copy of, or modify, this frame)"
            n97 = call <vilib>:"Add State(s) to Queue__jki_lib_state_machine.vi"("State(s) in (\"\")"=w295) -> ("States Out"=w294:string)  [unwired: 14 in]
          }
          frame "Process: Sync" {
            n98 = Unbundle By Name(w303) -> ("Self Reference"=w299:refnum<class "SMO.Control Experiment.lvclass">)
            n99 = call <vilib>:"WaitOnProcessSync.vi"("error in (no error)"=w298, "SMO"=w299) -> ("error out"=w297:errorcluster, "Don't run?"=w302:bool)  [unwired: 7 in, 1 out]
            n100 = Select(t="Data: Cleanup\nEvents: Unregister\nExit", s=w302, f="") -> (s? t:f=w296:string)
            n101 = call <vilib>:"Add State(s) to Queue__jki_lib_state_machine.vi"("State(s) in Front (\"\")"=w296, "State(s) in (\"\")"=w306) -> ("States Out"=w305:string)  [unwired: 13 in]
          }
          frame "---------- Events ----------" {
            # "Template Separator\n(You can make a copy of, or modify, this frame)"
            n102 = call <vilib>:"Add State(s) to Queue__jki_lib_state_machine.vi"("State(s) in (\"\")"=w311) -> ("States Out"=w310:string)  [unwired: 14 in]
          }
          frame "Events: Register" {
            # "Expand to add\nmore events"
            n103 = Unbundle By Name(w316) -> ("Self Reference"=w315:refnum<class "SMO.Control Experiment.lvclass">)
            n104 = call <vilib>:"GetProtectedEvents.vi"("SMO"=w315) -> ("error out"=w317:errorcluster, "SMO Protected Events"=w321:T27, "SMO out"=w314:refnum<class "SMO.Control Experiment.lvclass">)  [unwired: 8 in]
            n105 = call "SMO.Control Experiment.GetPrivateEvents.vi"("Control Experiment"=w314) -> ("error out"=w312:errorcluster, "Private Events"=w313:T28)  [unwired: 8 in, 1 out]
            n106 = register-events(w321, w313) -> (reference out=w322:refnum<event-registration>, error out=w318:errorcluster)  [unwired: 2 in]
            n107 = Merge Errors(w312, w320, w318, w317) -> (w319:errorcluster)
            n108 = call <vilib>:"Add State(s) to Queue__jki_lib_state_machine.vi"("State(s) in (\"\")"=w324) -> ("States Out"=w323:string)  [unwired: 14 in]
          }
          frame "Events: Unregister" {
            n109 = Unregister For Events(event registration refnum=w327, error in=w326) -> (error out=w325:errorcluster)
            n110 = call <vilib>:"Clear Errors.vi"("error in (no error)"=w325) -> ()  [unwired: 5 in, 2 out]
            n111 = call <vilib>:"Add State(s) to Queue__jki_lib_state_machine.vi"("State(s) in (\"\")"=w330) -> ("States Out"=w329:string)  [unwired: 14 in]
          }
          frame "---------- Configuration ----------" {
            n112 = call <vilib>:"Add State(s) to Queue__jki_lib_state_machine.vi"("State(s) in (\"\")"=w335) -> ("States Out"=w334:string)  [unwired: 14 in]
          }
          frame "Configuration: Initialize" {
            w350 = T29 3 items=["User Home"=0, "User Desktop"=1, "User Documents"=2, "User Application Data"=3, "User Preferences"=4, "User Temporary"=5, "Public Documents"=6, "Public Application Data"=7, "Public Preferences"=8, "Public Cache"=13, "System Core Libraries"=9, "System Installed Libraries"=10, "Application Files"=11, "Boot Volume Root"=12] ("system directory type")
            n113 = call <vilib>:"Get System Directory.vi"("system directory type"=w350) -> ("system directory"=w349:path)  [unwired: 10 in]
            n114 = Format Into String(format string="configuration_%s.ini", error in=w341, w339) -> (resulting string=w343:string, error out=w346:errorcluster)  [unwired: 1 in]
            n115 = Build Path(base path=w349, name or relative path="LevyLab\\Control Experiment UI") -> (appended path=w342:path)
            n116 = call <userlib>:"Create Dir if Non-Existant__ogtk.vi"("error in (no error)"=w346, "Directory Path"=w342) -> ("error out"=w345:errorcluster, "dup Directory Path"=w344:path)  [unwired: 7 in, 1 out]
            n117 = call <userlib>:"Write Path.vi"("error in (no error)"=w345, "Filename [Configuration.ini]"=w343, "Path"=w344) -> ("error out"=w340:errorcluster, "Configuration out"=w336:refnum<class "Configuration.lvclass">)  [unwired: 7 in]
            n118 = Bundle By Name(cluster=w338, "Config"=w336) -> (w337:T25)
            n119 = call <vilib>:"Add State(s) to Queue__jki_lib_state_machine.vi"("State(s) in (\"\")"=w353) -> ("States Out"=w352:string)  [unwired: 14 in]
          }
          frame "Configuration: Read File" {
            # "send to UI"
            n120 = Unbundle By Name(w359) -> ("Self Reference"=w354:refnum<class "SMO.Control Experiment.lvclass">, "UI Config"=w364:T10, "Config"=w363:refnum<class "Configuration.lvclass">)
            n121 = call <userlib>:"Read Configuration.vi"("INI Fomatted Cluster Type"=w364, "error in (no error)"=w360, "Configuration in"=w363) -> ("error out"=w361:errorcluster, "Configuration"=w362:variant)  [unwired: 6 in, 1 out]
            n122 = Variant To Data(error in=w361, type=w364, Variant=w362) -> (data=w357:T10, error out=w356:errorcluster)
            n123 = call "SMO.Control Experiment.getUIconfig.vi"("error in (no error)"=w356, "UI Configuration"=w357, "Control Experiment"=w354) -> ("error out"=w355:errorcluster)  [unwired: 7 in, 1 out]
            n124 = Bundle By Name(cluster=w359, "UI Config"=w357) -> (w358:T25)
            n125 = call <vilib>:"Add State(s) to Queue__jki_lib_state_machine.vi"("State(s) in (\"\")"=w367) -> ("States Out"=w366:string)  [unwired: 14 in]
          }
          frame "Configuration: Write File" {
            n126 = Unbundle By Name(w370) -> ("Config"=w372:refnum<class "Configuration.lvclass">, "UI Config"=w371:T10)
            n127 = call <userlib>:"Write Configuration.vi"("error in (no error)"=w369, "Variant"=w371, "Configuration in"=w372) -> ("error out"=w368:errorcluster)  [unwired: 7 in, 1 out]
            n128 = call <vilib>:"Add State(s) to Queue__jki_lib_state_machine.vi"("State(s) in (\"\")"=w375) -> ("States Out"=w374:string)  [unwired: 14 in]
          }
          frame "---------- KH ----------" {
            n129 = call <vilib>:"Add State(s) to Queue__jki_lib_state_machine.vi"("State(s) in (\"\")"=w380) -> ("States Out"=w379:string)  [unwired: 14 in]
          }
          frame "KH: Get Installed Shunt Resistor" {
            n130 = call <vilib>:"Add State(s) to Queue__jki_lib_state_machine.vi"("State(s) in (\"\")"=w385) -> ("States Out"=w384:string)  [unwired: 14 in]
          }
          frame "---------- Metadata ----------" {
            n131 = Unbundle By Name(w387) -> ("Config"=w386:refnum<class "Configuration.lvclass">)
            n132 = Bundle By Name(cluster=w387, "Config"=w386) -> (w388:T25)
            n133 = call <vilib>:"Add State(s) to Queue__jki_lib_state_machine.vi"("State(s) in (\"\")"=w392) -> ("States Out"=w391:string)  [unwired: 14 in]
          }
          frame "Metadata: Set Experiment" {
            n134 = Unbundle By Name(w407) -> ("C.E."=w403:refnum<class "Control Experiment.lvclass">, "UI Config"=w399:T10)
            n135 = Unbundle By Name(w399) -> ("Metadata.Username"=w397:string, "Metadata.Sample (SAXXXX)"=w396:string, "Metadata.Device (YYYYMMDD)"=w393:string, "Metadata.Description"=w394:string, "Instruments.Instrument"=w398:T5)
            n136 = call "Device ID.vi"("Date (YYYYMMDD)"=w393, "Sample (SAXXXX)"=w396) -> ("Device ID"=w395:string)  [unwired: 3 in]
            n137 = Bundle By Name(cluster=T4 {"User"="", "Device"="", "Device Path"=path "", "Device Description"="", "Experiment Path"=path "", "Experiment Description"="", "Instrument"=enum."MNK", "Instruments"=[], "Sweep"=[{"key"="OFF", "value"=variant}, {"key"="OFF", "value"=variant}, {"key"="OFF", "value"=variant}, {"key"="OFF", "value"=variant}]} ("Experiment Description"), "User"=w397, "Device"=w395, "Device Description"=w394, "Instrument"=w398) -> (w404:T4)
            n138 = call "Write Experiment Description (cluster).vi"("error in (no error)"=w401, "Experiment Description"=w404, "Control Experiment in"=w403) -> ("error out"=w400:errorcluster, "Control Experiment out"=w402:refnum<class "Control Experiment.lvclass">)  [unwired: 7 in]
            n139 = Bundle By Name(cluster=w407, "C.E."=w402) -> (w406:T25)
            n140 = call <vilib>:"Add State(s) to Queue__jki_lib_state_machine.vi"("State(s) in (\"\")"=w410) -> ("States Out"=w409:string)  [unwired: 14 in]
          }
          frame "Metadata: Set Wiring" {
            n141 = Unbundle By Name(w417) -> ("C.E."=w416:refnum<class "Control Experiment.lvclass">, "UI Config.UI Channels []"=w412:T11[])
            n142 = for {
              tunnel: w412 -> [w441] mode=indexing
              tunnel: [w440] -> w411 mode=indexing
              n143 = Unbundle By Name(w441) -> ("AI.Channel"=w424:u32, "AI.Gain"=w425:dbl, "Device.Electrode"=w426:string, "Device.Label"=w427:u16, "Device.Configuration"=w435:T14, "KH.Channel"=w433:u16, "KH.Configuration"=w438:T16, "KH.Gain"=w429:T17, "KH.Shunt Resistor"=w431:T18, "AO.Channel"=w423:u32, "AO.Gain"=w437:dbl)
              n144 = Format Into String(w427) -> (resulting string=w439:string)  [unwired: 3 in, 1 out]
              n145 = case shown="\"1000x\"" w429 {
                tunnel: [1 10 100 1000] -> w428
                frame "1x", Default {
                }
                frame "10x" {
                }
                frame "100x" {
                }
                frame "1000x" {
                }
              }
              n146 = case shown="\"Open\", Default" w431 {
                tunnel: [0 50 500 5000 50000 10000000] -> w430
                frame "Open", Default {
                }
                frame "50 Ohms" {
                }
                frame "500 Ohms" {
                }
                frame "5k Ohms" {
                }
                frame "50k Ohms" {
                }
                frame "10M Ohm" {
                }
              }
              n147 = Format Into String(w435) -> (resulting string=w436:string)  [unwired: 3 in, 1 out]
              n148 = Format Into String(w433) -> (resulting string=w434:string)  [unwired: 3 in, 1 out]
              n149 = Format Into String(w438) -> (resulting string=w432:string)  [unwired: 3 in, 1 out]
              n150 = Bundle By Name(cluster=T7 {"AI"={"Channel"=0, "Gain"=0.0}, "Device"={"Electrode"="", "Label"="", "Type"=""}, "KH"={"Channel"="", "Configuration"="", "Gain"=0, "Shunt Resistor"=0}, "AO"={"Channel"=0, "Gain"=0.0}} ("Wiring"), "AI.Channel"=w424, "AI.Gain"=w425, "Device.Electrode"=w426, "Device.Label"=w439, "Device.Type"=w436, "KH.Channel"=w434, "KH.Configuration"=w432, "KH.Gain"=w428, "KH.Shunt Resistor"=w430, "AO.Channel"=w423, "AO.Gain"=w437) -> (w440:T7)
            }
            n151 = call "Write Wiring Configuration v2.vi"("error in (no error)"=w414, "Wiring Configuration v2"=w411, "Control Experiment in"=w416) -> ("error out"=w413:errorcluster, "Control Experiment out"=w415:refnum<class "Control Experiment.lvclass">)  [unwired: 7 in]
            n152 = Bundle By Name(cluster=w417, "C.E."=w415) -> (w418:T25)
            n153 = call <vilib>:"Add State(s) to Queue__jki_lib_state_machine.vi"("State(s) in (\"\")"=w421) -> ("States Out"=w420:string)  [unwired: 14 in]
          }
          frame "Metadata: Set Data Path" {
            n154 = Unbundle By Name(w457) -> ("C.E."=w456:refnum<class "Control Experiment.lvclass">, "UI Config.Metadata.Default Path"=w452:path)
            n155 = call "Initialize Device Folder.vi"("error in (no error)"=w455, "Default Path in"=w452, "Control Experiment"=w456) -> ("error out"=w454:errorcluster, "Control Experiment out"=w453:refnum<class "Control Experiment.lvclass">)  [unwired: 6 in, 1 out]
            n156 = Bundle By Name(cluster=w457, "C.E."=w453) -> (w458:T25)
            n157 = call <vilib>:"Add State(s) to Queue__jki_lib_state_machine.vi"("State(s) in (\"\")"=w461) -> ("States Out"=w460:string)  [unwired: 14 in]
          }
          frame "Metadata: Update Comments" {
            n158 = Unbundle By Name(w468) -> ("C.E."=w466:refnum<class "Control Experiment.lvclass">)
            n159 = call "Generate Comments.vi"("error in (no error)"=w463, "Control Experiment"=w466) -> ("error out"=w464:errorcluster, "Control Experiment out"=w465:refnum<class "Control Experiment.lvclass">)  [unwired: 6 in, 1 out]
            n160 = call <vilib>:"Clear Errors.vi"("error in (no error)"=w464, "specific error code to clear (0: all)"=63) -> ("error out"=w462:errorcluster)  [unwired: 4 in, 1 out]
            n161 = Bundle By Name(cluster=w468, "C.E."=w465) -> (w469:T25)
            n162 = call <vilib>:"Add State(s) to Queue__jki_lib_state_machine.vi"("State(s) in (\"\")"=w472) -> ("States Out"=w471:string)  [unwired: 14 in]
          }
          frame "Metadata: Set Device JSON" {
            w492 = T30 {"Device"={"Device"="", "User"="", "Time"="", "Computer Name"=""}, "Wiring"={"Lockin Ch"=[], "KH Electrodes"=[], "KH Labels"=[], "Other Electrodes"=[], "Other Labels"=[]}}  # Control Experiment JSON
            n163 = Unbundle By Name(w493) -> ("C.E."=w473:refnum<class "Control Experiment.lvclass">, "UI Config"=w490:T10)
            n164 = flat-sequence {
              tunnel: [string[] [] ("Wiring.KH Electrodes")] -> w480
              tunnel: [u32[] [] ("Wiring.Lockin Ch")] -> w481
              tunnel: w479 -> [_]
              frame #0 {
                # "something to dot/gv"
              }
            }
            n165 = Unbundle By Name(w490) -> ("Metadata.Sample (SAXXXX)"=w485:string, "Metadata.Device (YYYYMMDD)"=w487:string, "Metadata.Username"=w486:string, "UI Channels []"=w479:T11[])
            n166 = call "Get Date Time ISO.vi"("error in (no error)"=w483) -> ("error out"=w482:errorcluster, "ISO 8601 date-time string"=w489:string)  [unwired: 8 in, 1 out]
            n167 = call "Device ID.vi"("Date (YYYYMMDD)"=w487, "Sample (SAXXXX)"=w485) -> ("Device ID"=w484:string)  [unwired: 3 in]
            n168 = call "Get Computer Name.vi"("error in (no error)"=w482) -> ("error out"=w478:errorcluster, "name"=w488:string)  [unwired: 9 in]
            n169 = Bundle By Name(cluster=w492, "Device.Device"=w484, "Device.User"=w486, "Device.Time"=w489, "Device.Computer Name"=w488, "Wiring.Lockin Ch"=w481, "Wiring.KH Electrodes"=w480, "Wiring.KH Labels"=w480, "Wiring.Other Electrodes"=w480, "Wiring.Other Labels"=w480) -> (w491:T30)
            n170 = call "To JSON Text.vim"("error in (no error)"=w478, "Anything"=w491) -> ("error out"=w476:errorcluster, "<JSON>"=w477:string)  [unwired: 8 in]
            n171 = call "Write json.vi"("error in (no error)"=w476, "json"=w477, "Control Experiment in"=w473) -> ("error out"=w475:errorcluster, "Control Experiment out"=w474:refnum<class "Control Experiment.lvclass">)  [unwired: 7 in]
            n172 = Bundle By Name(cluster=w493, "C.E."=w474) -> (w494:T25)
            n173 = call <vilib>:"Add State(s) to Queue__jki_lib_state_machine.vi"("State(s) in (\"\")"=w497) -> ("States Out"=w496:string)  [unwired: 14 in]
          }
          frame "---------- C.E. ----------" {
            n174 = Unbundle By Name(w501) -> ("Self Reference"=w500:refnum<class "SMO.Control Experiment.lvclass">)
            n175 = Bundle By Name(cluster=w501, "Self Reference"=w500) -> (w502:T25)
            n176 = call <vilib>:"Add State(s) to Queue__jki_lib_state_machine.vi"("State(s) in (\"\")"=w506) -> ("States Out"=w505:string)  [unwired: 14 in]
          }
          frame "C.E.: Initialize Instruments" {
            n177 = Unbundle By Name(w511) -> ("C.E."=w510:refnum<class "Control Experiment.lvclass">)
            n178 = call "Load Instrument Classes.vi"("error in (no error)"=w508, "Control Experiment.lvclass"=w510) -> ("error out"=w507:errorcluster, "Control Experiment out"=w509:refnum<class "Control Experiment.lvclass">)  [unwired: 8 in]
            n179 = Bundle By Name(cluster=w511, "C.E."=w509) -> (w512:T25)
            n180 = call <vilib>:"Add State(s) to Queue__jki_lib_state_machine.vi"("State(s) in (\"\")"=w515) -> ("States Out"=w514:string)  [unwired: 14 in]
          }
          frame "C.E.: Open Krohn Hite" {
            n181 = Unbundle By Name(w529) -> ("C.E."=w528:refnum<class "Control Experiment.lvclass">, "UI Config"=w523:T10)
            n182 = call "Read Instruments.vi"("error in (no error)"=w522, "Control Experiment in"=w528) -> ("error out"=w521:errorcluster, "Instruments"=w519:T31, "Control Experiment out"=w525:refnum<class "Control Experiment.lvclass">)  [unwired: 7 in]
            n183 = Unbundle By Name(w523) -> ("Instruments.KH Addresses"=w517:refnum<visa-resource-name>[])
            n184 = Unbundle By Name(w519) -> ("KH7008"=w518:refnum<class "Instrument.KH7008.lvclass">[])
            n185 = for {
              tunnel: [w539] -> w520 mode=indexing
              tunnel: w521 -> [w538]
              tunnel: [w537] -> w516
              tunnel: w517 -> [w536] mode=indexing
              tunnel: w518 -> [w535]
              n186 = Index Array(array=w535) -> (element=w534:refnum<class "Instrument.KH7008.lvclass">)  [unwired: 1 in]
              n187 = call-dynamic "Open.vi"("error in (no error)"=w538, "address"=w536, "Instrument.KH7008 in"=w534) -> ("error out"=w537:errorcluster, "Instrument.KH7008 out"=w539:refnum<class "Instrument.KH7008.lvclass">)  [unwired: 7 in]
            }
            n188 = Bundle By Name(cluster=w519, "KH7008"=w520) -> (w526:T31)
            n189 = call "Write Instruments.vi"("error in (no error)"=w516, "Instruments"=w526, "Control Experiment in"=w525) -> ("error out"=w524:errorcluster, "Control Experiment out"=w527:refnum<class "Control Experiment.lvclass">)  [unwired: 7 in]
            n190 = Bundle By Name(cluster=w529, "C.E."=w527) -> (w530:T25)
            n191 = call <vilib>:"Add State(s) to Queue__jki_lib_state_machine.vi"("State(s) in (\"\")"=w533) -> ("States Out"=w532:string)  [unwired: 14 in]
          }
          frame "C.E.: Initialize KH Cluster" {
            n192 = Unbundle By Name(w551) -> ("UI Config"=w540:T10)
            n193 = Unbundle By Name(w540) -> ("Instruments.KH Addresses"=w541:refnum<visa-resource-name>[], "Krohn Hite.Bandwidth Filter"=w546:T21, "Krohn Hite.Coupling"=w547:T20)
            n194 = call "Initialize KH Cluster.vi"("error in (no error)"=w543, "KH Addresses"=w541) -> ("error out"=w545:errorcluster, "KH Cluster out"=w550:T22)  [unwired: 8 in]
            n195 = call "Set KH BW Filter.vi"("error in (no error)"=w545, "Bandwidth Filter"=w546, "KH Cluster"=w550) -> ("error out"=w544:errorcluster, "KH Cluster out"=w549:T22)  [unwired: 7 in]
            n196 = call "Set KH Coupling.vi"("error in (no error)"=w544, "Coupling"=w547, "KH Cluster"=w549) -> ("error out"=w542:errorcluster, "KH Cluster out"=w548:T22)  [unwired: 7 in]
            n197 = Bundle By Name(cluster=w551, "KH Cluster"=w548) -> (w552:T25)
            n198 = call <vilib>:"Add State(s) to Queue__jki_lib_state_machine.vi"("State(s) in (\"\")"=w555) -> ("States Out"=w554:string)  [unwired: 14 in]
          }
          frame "C.E.: Get SR Type" {
            # "send back to UI"
            n199 = Unbundle By Name(w562) -> ("Self Reference"=w559:refnum<class "SMO.Control Experiment.lvclass">, "UI Config"=w561:T10)
            n200 = Unbundle By Name(w561) -> ("Instruments.KH Addresses"=w564:refnum<visa-resource-name>[])
            n201 = Index Array(array=w564) -> (element=w560:refnum<visa-resource-name>)  [unwired: 1 in]
            n202 = call <userlib>:"Shunt - Check 500 or 10M.vi"("error in (no error)"=w563, "VISA Refnum in"=w560) -> ("error out"=w557:errorcluster, "SR"=w558:enum16{"500", "10M"})  [unwired: 7 in, 1 out]
            n203 = call "SMO.Control Experiment.getKHShuntType.vi"("error in (no error)"=w557, "getKHShuntType"=w558, "Control Experiment"=w559) -> ("error out"=w556:errorcluster)  [unwired: 7 in, 1 out]
            n204 = call <vilib>:"Add State(s) to Queue__jki_lib_state_machine.vi"("State(s) in (\"\")"=w567) -> ("States Out"=w566:string)  [unwired: 14 in]
          }
          frame "C.E.: Set Krohn Hite" {
            n205 = Unbundle By Name(w589) -> ("C.E."=w577:refnum<class "Control Experiment.lvclass">, "KH Cluster"=w569:T22, "UI Config"=w576:T10)
            n206 = Unbundle By Name(w576) -> ("UI Channels []"=w574:T11[], "Number of AI"=w573:i32, "UI Channels []"=w568:T11[])
            n207 = call "Read Instruments.vi"("error in (no error)"=w571, "Control Experiment in"=w577) -> ("error out"=w570:errorcluster, "Instruments"=w587:T31)  [unwired: 7 in, 1 out]
            n208 = Unbundle By Name(w587) -> ("Lockin"=w584:refnum<class "Instrument.Lockin.lvclass">, "KH7008"=w588:refnum<class "Instrument.KH7008.lvclass">[])
            n209 = call "Set KH Cluster From UI Array.vi"("error in (no error)"=w570, "Number of AI"=w573, "UI Channels []"=w574, "KH Cluster"=w569) -> ("error out"=w572:errorcluster, "KH Cluster out"=w575:T22)  [unwired: 6 in]
            n210 = for {
              tunnel: w572 -> [w605]
              tunnel: [w598] -> w580
              tunnel: w575 -> [w604] mode=indexing
              tunnel: w588 -> [w603] mode=indexing
              tunnel: [w597] -> w585 mode=concatenating
              n211 = Unbundle(w604) -> ("KH Ch Array"=w596:T23[])  [unwired: 1 out]
              n212 = call <userlib>:"Write Channel Setting.vi"("error in (no error)"=w605, "Channel Setting"=w596, "KH7008 in"=w603) -> ("error out"=w601:errorcluster, "KH7008 out"=w602:refnum<class "Instrument.KH7008.lvclass">)  [unwired: 7 in]
              n213 = call <userlib>:"KH Control.vi"("error in"=w601, "KH7008"=w602) -> ("error out"=w600:errorcluster, "KH7008.lvclass out"=w599:refnum<class "Instrument.KH7008.lvclass">)  [unwired: 8 in]
              n214 = call <userlib>:"Read Gain.vi"("error in (no error)"=w600, "KH7008 in"=w599) -> ("error out"=w598:errorcluster, "Gain"=w597:dbl[])  [unwired: 7 in, 1 out]
            }
            n215 = for {
              tunnel: w568 -> [w595] mode=indexing
              tunnel: [w594] -> w583 mode=indexing
              tunnel: [w593] -> w579 mode=indexing
              n216 = Unbundle By Name(w595) -> ("AI.Gain"=w594:dbl, "AO.Gain"=w593:dbl)
            }
            n217 = call "Multiply Gains.vi"("Other Gain"=w583, "Gain"=w585) -> ("Gain x Other Gain"=w586:dbl[])
            n218 = call <userlib>:"setInputGain.vi"("error in (no error)"=w580, "InputGain"=w586, "Instrument.Lockin in"=w584) -> ("error out"=w582:errorcluster, "Instrument.Lockin out"=w581:refnum<class "Instrument.Lockin.lvclass">)  [unwired: 7 in]
            n219 = call <userlib>:"setOutputGain.vi"("error in (no error)"=w582, "OutputGain"=w579, "Instrument.Lockin in"=w581) -> ("error out"=w578:errorcluster)  [unwired: 7 in, 1 out]
            n220 = call <vilib>:"Add State(s) to Queue__jki_lib_state_machine.vi"("State(s) in (\"\")"=w592) -> ("States Out"=w591:string)  [unwired: 14 in]
          }
          frame "C.E.: Open Lockin" {
            n221 = Unbundle By Name(w619) -> ("C.E."=w618:refnum<class "Control Experiment.lvclass">, "UI Config"=w612:T10)
            n222 = call "Read Instruments.vi"("error in (no error)"=w611, "Control Experiment in"=w618) -> ("error out"=w610:errorcluster, "Instruments"=w607:T31, "Control Experiment out"=w615:refnum<class "Control Experiment.lvclass">)  [unwired: 7 in]
            n223 = Unbundle By Name(w612) -> ("Instruments.Lockin Address"=w613:string)
            n224 = Unbundle By Name(w607) -> ("Lockin"=w606:refnum<class "Instrument.Lockin.lvclass">)
            n225 = call-dynamic "Open.vi"("error in (no error)"=w610, "address"=w613, "Instrument.Lockin in"=w606) -> ("error out"=w609:errorcluster, "Instrument.Lockin out"=w608:refnum<class "Instrument.Lockin.lvclass">)  [unwired: 7 in]
            n226 = Bundle By Name(cluster=w607, "Lockin"=w608) -> (w616:T31)
            n227 = call "Write Instruments.vi"("error in (no error)"=w609, "Instruments"=w616, "Control Experiment in"=w615) -> ("error out"=w614:errorcluster, "Control Experiment out"=w617:refnum<class "Control Experiment.lvclass">)  [unwired: 7 in]
            n228 = Bundle By Name(cluster=w619, "C.E."=w617) -> (w620:T25)
            n229 = call <vilib>:"Add State(s) to Queue__jki_lib_state_machine.vi"("State(s) in (\"\")"=w623) -> ("States Out"=w622:string)  [unwired: 14 in]
          }
          frame "C.E.: Open Strain Cell" {
            n230 = Unbundle By Name(w637) -> ("C.E."=w636:refnum<class "Control Experiment.lvclass">, "UI Config"=w630:T10)
            n231 = call "Read Instruments.vi"("error in (no error)"=w629, "Control Experiment in"=w636) -> ("error out"=w628:errorcluster, "Instruments"=w625:T31, "Control Experiment out"=w633:refnum<class "Control Experiment.lvclass">)  [unwired: 7 in]
            n232 = Unbundle By Name(w630) -> ("Instruments.Strain Cell Address"=w631:refnum<visa-resource-name>)
            n233 = Unbundle By Name(w625) -> ("Strain Cell"=w624:refnum<class "Instrument.Strain.lvclass">)
            n234 = call-dynamic "Open.vi"("error in (no error)"=w628, "address"=w631, "Instrument in"=w624) -> ("error out"=w627:errorcluster, "Instrument out"=w626:refnum<class "Instrument.Strain.lvclass">)  [unwired: 7 in]
            n235 = Bundle By Name(cluster=w625, "Strain Cell"=w626) -> (w634:T31)
            n236 = call "Write Instruments.vi"("error in (no error)"=w627, "Instruments"=w634, "Control Experiment in"=w633) -> ("error out"=w632:errorcluster, "Control Experiment out"=w635:refnum<class "Control Experiment.lvclass">)  [unwired: 7 in]
            n237 = Bundle By Name(cluster=w637, "C.E."=w635) -> (w638:T25)
            n238 = call <vilib>:"Add State(s) to Queue__jki_lib_state_machine.vi"("State(s) in (\"\")"=w641) -> ("States Out"=w640:string)  [unwired: 14 in]
          }
          frame "C.E.: Open C Bridge" {
            n239 = Unbundle By Name(w655) -> ("C.E."=w654:refnum<class "Control Experiment.lvclass">, "UI Config"=w648:T10)
            n240 = Unbundle By Name(w648) -> ("Instruments.Capacitance Bridge Address"=w649:refnum<visa-resource-name>)
            n241 = call "Read Instruments.vi"("error in (no error)"=w647, "Control Experiment in"=w654) -> ("error out"=w646:errorcluster, "Instruments"=w643:T31, "Control Experiment out"=w651:refnum<class "Control Experiment.lvclass">)  [unwired: 7 in]
            n242 = Unbundle By Name(w643) -> ("Capacitance Bridge"=w642:refnum<class "Instrument.CBridge.lvclass">)
            n243 = call-dynamic "Open.vi"("error in (no error)"=w646, "address"=w649, "Instrument in"=w642) -> ("error out"=w645:errorcluster, "Instrument out"=w644:refnum<class "Instrument.CBridge.lvclass">)  [unwired: 7 in]
            n244 = Bundle By Name(cluster=w643, "Capacitance Bridge"=w644) -> (w652:T31)
            n245 = call "Write Instruments.vi"("error in (no error)"=w645, "Instruments"=w652, "Control Experiment in"=w651) -> ("error out"=w650:errorcluster, "Control Experiment out"=w653:refnum<class "Control Experiment.lvclass">)  [unwired: 7 in]
            n246 = Bundle By Name(cluster=w655, "C.E."=w653) -> (w656:T25)
            n247 = call <vilib>:"Add State(s) to Queue__jki_lib_state_machine.vi"("State(s) in (\"\")"=w659) -> ("States Out"=w658:string)  [unwired: 14 in]
          }
          frame "C.E.: Write XML" {
            n248 = Unbundle By Name(w665) -> ("C.E."=w663:refnum<class "Control Experiment.lvclass">)
            n249 = call "Control Experiment FGV.vi"("Function"=enum16{"read", "write"}."write", "error in (no error)"=w661, "Control Experiment.lvclass"=w663) -> ("error out"=w660:errorcluster, "Control Experiment.lvclass out"=w662:refnum<class "Control Experiment.lvclass">)  [unwired: 7 in]
            n250 = Bundle By Name(cluster=w665, "C.E."=w662) -> (w666:T25)
            n251 = call <vilib>:"Add State(s) to Queue__jki_lib_state_machine.vi"("State(s) in (\"\")"=w669) -> ("States Out"=w668:string)  [unwired: 14 in]
          }
          frame "C.E.: Write PGSQL" {
            w670 = FALSE  # finished taking data
            w687 = ""
            n252 = Unbundle By Name(w688) -> ("Self Reference"=w685:refnum<class "SMO.Control Experiment.lvclass">, "UI Config"=w683:T10)
            n253 = Unbundle By Name(w683) -> ("Instruments.Instrument"=w678:T5, "Metadata.Sample (SAXXXX)"=w682:string, "Metadata.Device (YYYYMMDD)"=w673:string, "Metadata.Username"=w672:string)
            n254 = call "Device ID.vi"("Date (YYYYMMDD)"=w673, "Sample (SAXXXX)"=w682) -> ("Device ID"=w671:string)  [unwired: 3 in]
            n255 = call "Device and User PGSQL Paths.vi"("instrument"=w678) -> ("User Path"=w676:string, "Device Path"=w677:string)  [unwired: 5 in]
            n256 = Select(t=w687, s=w670, f=w671) -> (s? t:f=w675:string)
            n257 = Select(t=w687, s=w670, f=w672) -> (s? t:f=w674:string)
            n258 = call <userlib>:"Instrument.LogPGSQL.vi"("error in (no error)"=w681, "Data"=w675, "Path"=w677, "Instrument"=w685) -> ("error out"=w679:errorcluster, "Instrument out"=w686:refnum<class "SMO.Control Experiment.lvclass">)  [unwired: 6 in]
            n259 = call <userlib>:"Instrument.LogPGSQL.vi"("error in (no error)"=w679, "Data"=w674, "Path"=w676, "Instrument"=w686) -> ("error out"=w680:errorcluster, "Instrument out"=w684:refnum<class "SMO.Control Experiment.lvclass">)  [unwired: 6 in]
            n260 = Bundle By Name(cluster=w688, "Self Reference"=w684) -> (w689:T25)
            n261 = call <vilib>:"Add State(s) to Queue__jki_lib_state_machine.vi"("State(s) in (\"\")"=w692) -> ("States Out"=w691:string)  [unwired: 14 in]
          }
        }
      }
    }
    frame Error {
    }
  }
  n262 = call-parent "Process.vi"("error in"=w5, "Instrument"=w4) -> ("error out"=w2:errorcluster, "Instrument out"=→"Control Experiment out":refnum<class "SMO.Control Experiment.lvclass">)  [unwired: 8 in]
  n263 = Merge Errors(w2, w1) -> (→"error out":errorcluster)
